vi "Omniax_mDrive_R_2016.vi"() -> ()   [LabVIEW 2014]
uses:
  <vilib>/Utility/file.llb/Read From Spreadsheet File (I64).vi
  <vilib>/Utility/file.llb/Read From Spreadsheet File (string).vi
  <vilib>/Instr/_visa.llb/VISA Configure Serial Port (Instr).vi
  <vilib>/Utility/file.llb/Write To Spreadsheet File (I64).vi
  <vilib>/Utility/file.llb/Write To Spreadsheet File (string).vi
panel:
  in  "R Move Set":bool
  in  "SSE:OmniaxR.SV":dbl
  in  "X Position SP mm":dbl
  in  "X Velocity SP mm/sec":dbl
  in  "X Move Set":bool
  in  "Y Move Set":bool
  in  "Y Position SP mm":dbl
  in  "Y Velocity SP mm/sec":dbl
  in  "Z Position SP mm":dbl
  in  "Z Velocity SP mm/sec":dbl
  in  "Z Move Set":bool
  in  "Reset Y Position mm":dbl
  out "Reset Y Motor Steps":i32
  in  "Reset X Position mm":dbl
  out "Reset X Motor Steps":i32
  in  "Reset Z Position mm":dbl
  out "Reset Z Motor Steps":i32
  in  "Submit":bool
  in  "ELOG":string
  out "Z max step":i32
  in  "V5 position 15360000":i32
  out "R Velocity MVdeg/sec":dbl format="%.3f"
  out "R Position MV deg":dbl
  out "Z Velocity MV mm/sec":dbl format="%.3f"
  out "Z Position MV mm":dbl
  out "Y Velocity MV mm/sec":dbl format="%.3f"
  out "Y Position MV mm":dbl
  out "X Velocity MV mm/sec":dbl format="%.3f"
  out "X Position MV mm":dbl
  out "Presets":i32[][](array[numeric])
  in  "stop":bool
  in  "Tab Control 3":enum32{"Status", "Reset"}(tab)
  out "R in Range":bool
  out "R Scan":bool
  out "R in Motion":bool
  out "R Backlash corr":bool
  out "R Ready":bool
  in  "Reset R Position deg":dbl
  out "Reset R Motor Steps":i32
  in  "Reset":bool
  in  "Tab Control 2":enum32{"mm", "step"}(tab)
  in  "X Scan Length SP mm":dbl
  in  "X Scan Velocity SP mm/sec":dbl
  in  "X Scan set":bool
  in  "Y Scan Length SP mm":dbl
  in  "Y Scan Velocity SP mm/sec":dbl
  in  "Y Scan set":bool
  in  "Z Scan Length SP mm":dbl
  in  "Z Scan Velocity SP mm/sec":dbl
  in  "Z Scan set":bool
  in  "R Scan Length SP deg":dbl
  in  "R Scan Velocity SP deg/sec":dbl
  in  "R Scan set":bool
  in  "X Scan Velocity SP steps/sec":i32=1 min=1 max=102400 step=1
  in  "X Scan Length SP steps":i32 min=-2816000 max=1792000 step=100
  out "X Scan length MV mm":dbl
  out "X Scan velocity MV mm/sec":dbl format="%#_6f"
  in  "Y Scan Velocity SP steps/sec":i32=1 min=1 max=102400 step=1
  in  "Y Scan Length SP steps":i32 min=-1930240 max=2677760 step=100
  out "Y Scan length MV mm":dbl
  out "Y Scan velocity MV mm/sec":dbl format="%#_6f"
  in  "Z Scan Velocity SP steps/sec":i32=1 min=1 max=102400 step=1
  in  "Z Scan Length SP steps":i32 min=-91980800 max=10419200 step=100
  out "Z Scan length MV mm":dbl
  out "Z Scan velocity MV mm/sec":dbl format="%#_6f"
  in  "R Scan Velocity SP steps/sec":i32=1 min=1 max=102400 step=1
  in  "R Scan Length SP steps":i32 min=-1501867 max=10786133 step=100
  out "R Scan length MV deg":dbl
  out "R Scan velocity MV deg/sec":dbl format="%#_6f"
  out "atan Y/Z":dbl
  in  "Tab Control":enum32{"mm", "preset", "step"}(tab)
  in  "R Velocity SP deg/sec":dbl
  in  "Add Button":bool
  in  "String":string
  in  "Delete Button":bool
  in  "Preset positions":i32(ring) items=["ZERO", "Default", "CDOSE", "QMS", "test", "test2", "test3", "yag position", "Sample Long Edge  ", "SPUTTER POS"]
  in  "Set Button":bool
  in  "X Velocity SP step/sec":i32 min=1 max=128000
  in  "Y Velocity SP step/sec":i32 min=1 max=128000
  in  "Z Velocity SP step/sec":i32 min=1 max=204800
  in  "R Velocity SP step/sec":i32 min=1 max=10000
  in  "Y Step SP":i32=-20000 min=-2304000 max=2304000 step=500
  in  "X Step SP":i32=-20000 min=-2304000 max=2304000 step=500
  in  "Z Step SP":i32=-20000 min=0 max=102400000 step=500
  in  "R Step SP":i32=-20000 min=-61440000 max=61440000 step=500
  out "X Step PV":i32 max=2000
  out "Y Step PV":i32 max=2000
  out "Z Step PV":i32 max=2000
  out "R Step PV":i32 max=2000
  in  "Clear ZY":bool
  out "X Scan Duration":dbl
  out "Y Scan Duration":dbl
  out "Z Scan Duration":dbl
  out "R Scan Duration":dbl
  out "R Backlash steps/sec":i32
  out "R Backlash":i32
  out "R Holding Current %":i32
  out "R Run Current %":i32
  out "R offset deg":dbl
  out "R deg/rev":dbl
  out "R steps/rev":u32
  out "R velocity PV step/sec":i32
  out "R MINPOS":i32=-94296
  out "R MAXPOS":i32=-34296
  out "R COM PORT":refnum<visa-resource-name>="COM5"
  in  "R Scan OK":bool
  in  "R Go":bool
  out "R Position deg PV":dbl
  out "Z Backlash steps/sec":i32
  out "Z Backlash":i32
  out "Z Holding Current %":i32
  out "Z Run Current %":i32
  out "Z offset mm":dbl
  out "Z mm/rev":dbl
  out "Z steps/rev":u32
  out "Z  velocity PV step/sec":i32
  in  "Z Scan OK":bool
  in  "Z Go":bool
  out "Z Position mm PV":dbl
  out "X Position mm PV":dbl
  out "X velocity PV step/sec":i32
  in  "X Scan OK":bool
  in  "X Go":bool
  out "X Backlash steps/sec":i32
  out "X Backlash":i32
  out "X Holding Current %":i32
  out "X Run Current %":i32
  out "X offset mm":dbl
  out "X mm/rev":dbl
  out "X steps/rev":u32
  out "Y Backlash steps/sec":i32
  out "Y Backlash":i32
  out "Y Holding Current %":i32
  out "Y Run Current %":i32
  in  "Scan Cancel":bool
  out "Y Position mm PV":dbl
  out "Y offset mm":dbl
  out "Y mm/rev":dbl
  out "Y steps/rev":u32
  out "Y velocity PV step/sec":i32
  in  "Y Scan OK":bool
  in  "Scan Go":bool
  in  "Stop":bool
  in  "Y Go":bool
  # "COM13"
  # "Goto position"
  # "SSE:OmniaxR.RV"
  # "R"
  # "MX"
  # "MR"
  # "MY"
  # "MZ"
  # "L"
  # "M"
  # "B"
  # "S"
  # "R"
  # "Preset position"
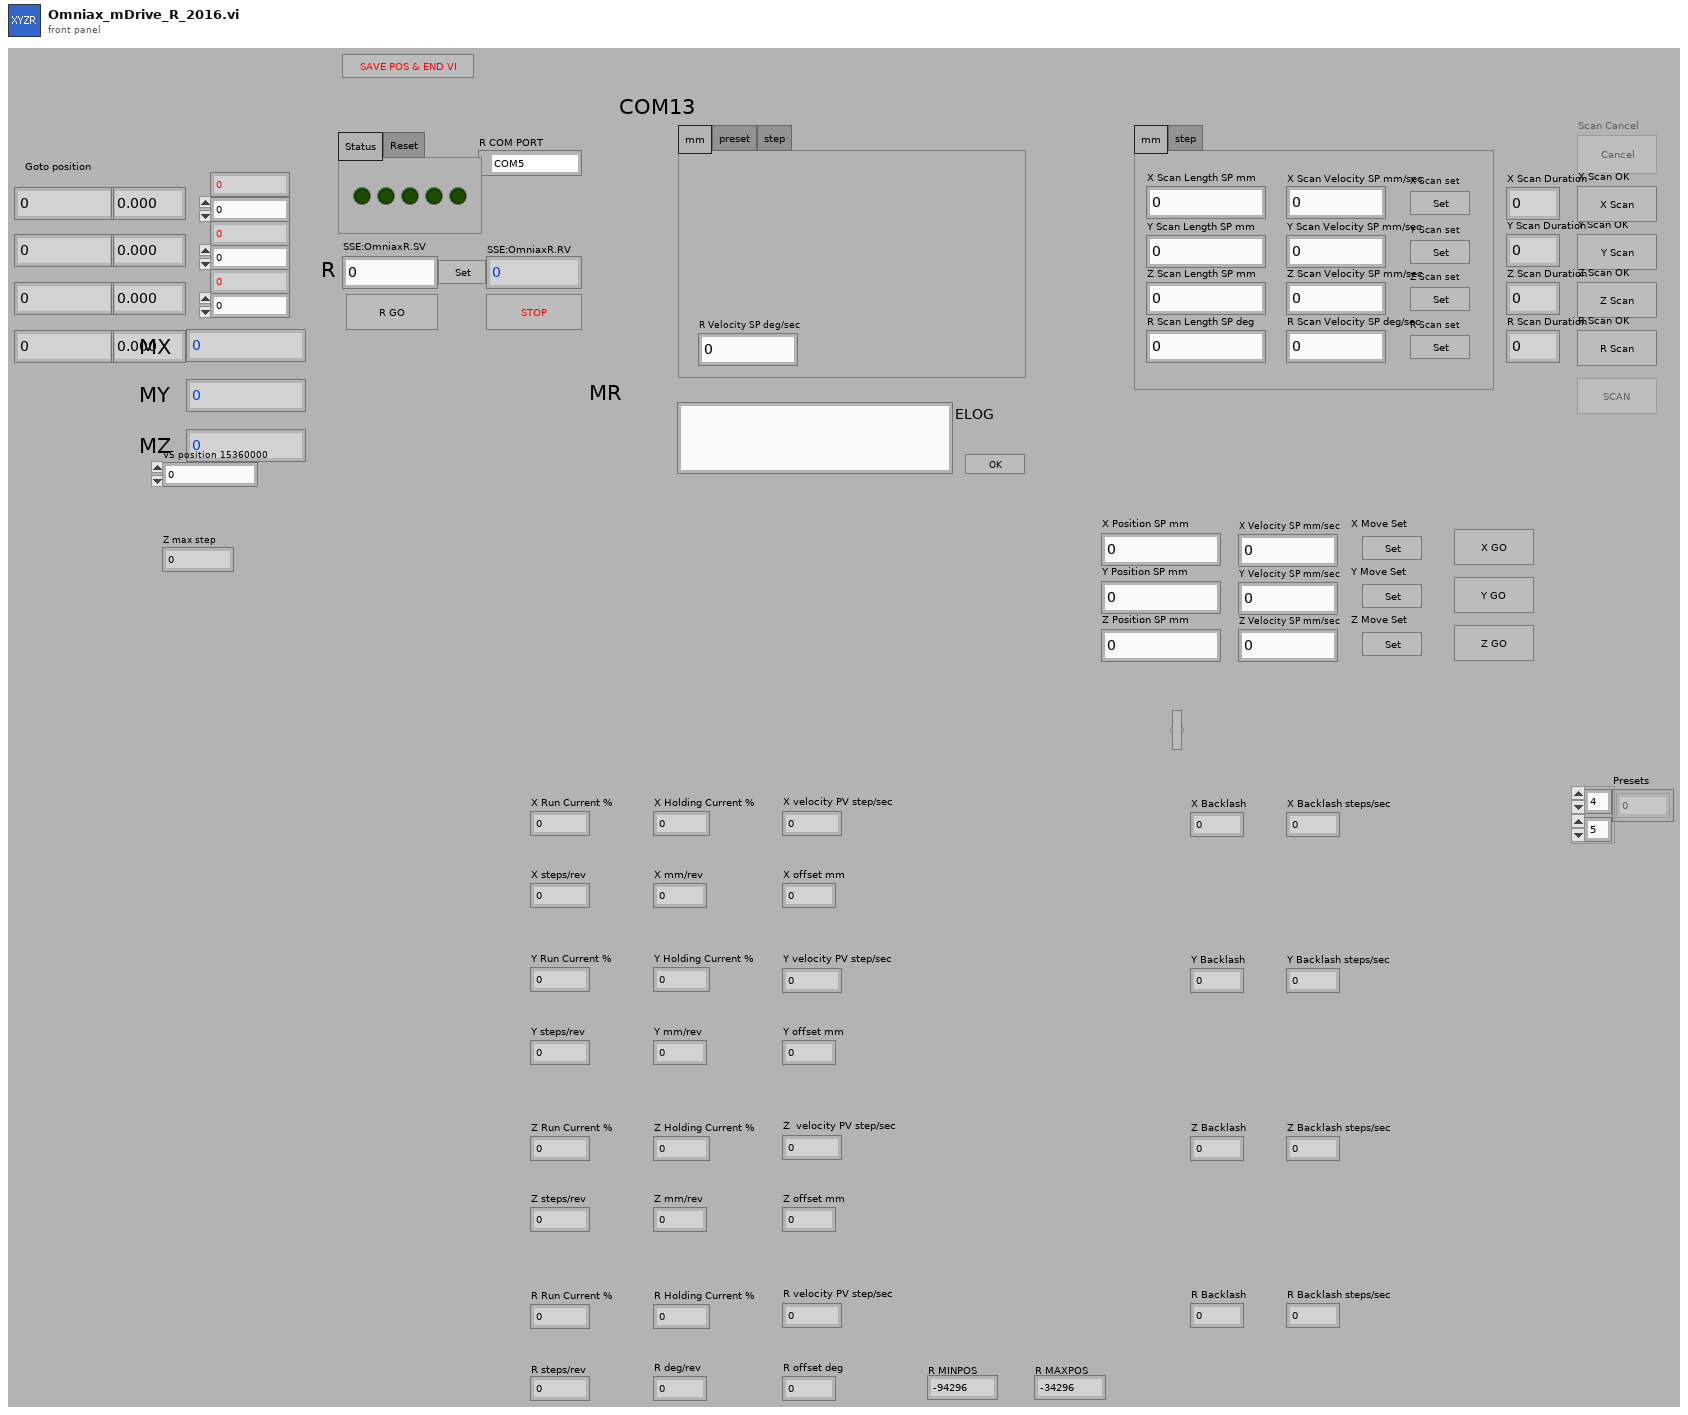
[diagram p1: front panel]
types:
  T1 = enum16{"Stop", "Reset", "Run Current", "Holding Current", "Accel Rate", "Decel Rate", "Move to Relative Position", "Move to Absolute Position", "Echo Mode", "Print Parameter", "Send String", "Microstep Resolution", "Set Current Position", "Max Velocity"}
  T2 = enum8{"Enabled", "Disabled", "Disabled and Grayed Out"}
  T3 = cluster{"first row[0]":i64, "first row[1]":i64, "first row[2]":i64, "first row[3]":i64, "first row[4]":i64, "first row[5]":i64, "first row[6]":i64, "first row[7]":i64, "first row[8]":i64}
  T4 = enum16{"open", "replace", "create", "open or create", "replace or create", "replace or create with confirmation"}
  T5 = cluster{"Value[0]":i32, "Value[1]":i32, "Value[2]":i32, "Value[3]":i32, "Value[4]":i32, "Value[5]":i32, "Value[6]":i32, "Value[7]":i32, "Value[8]":i32}
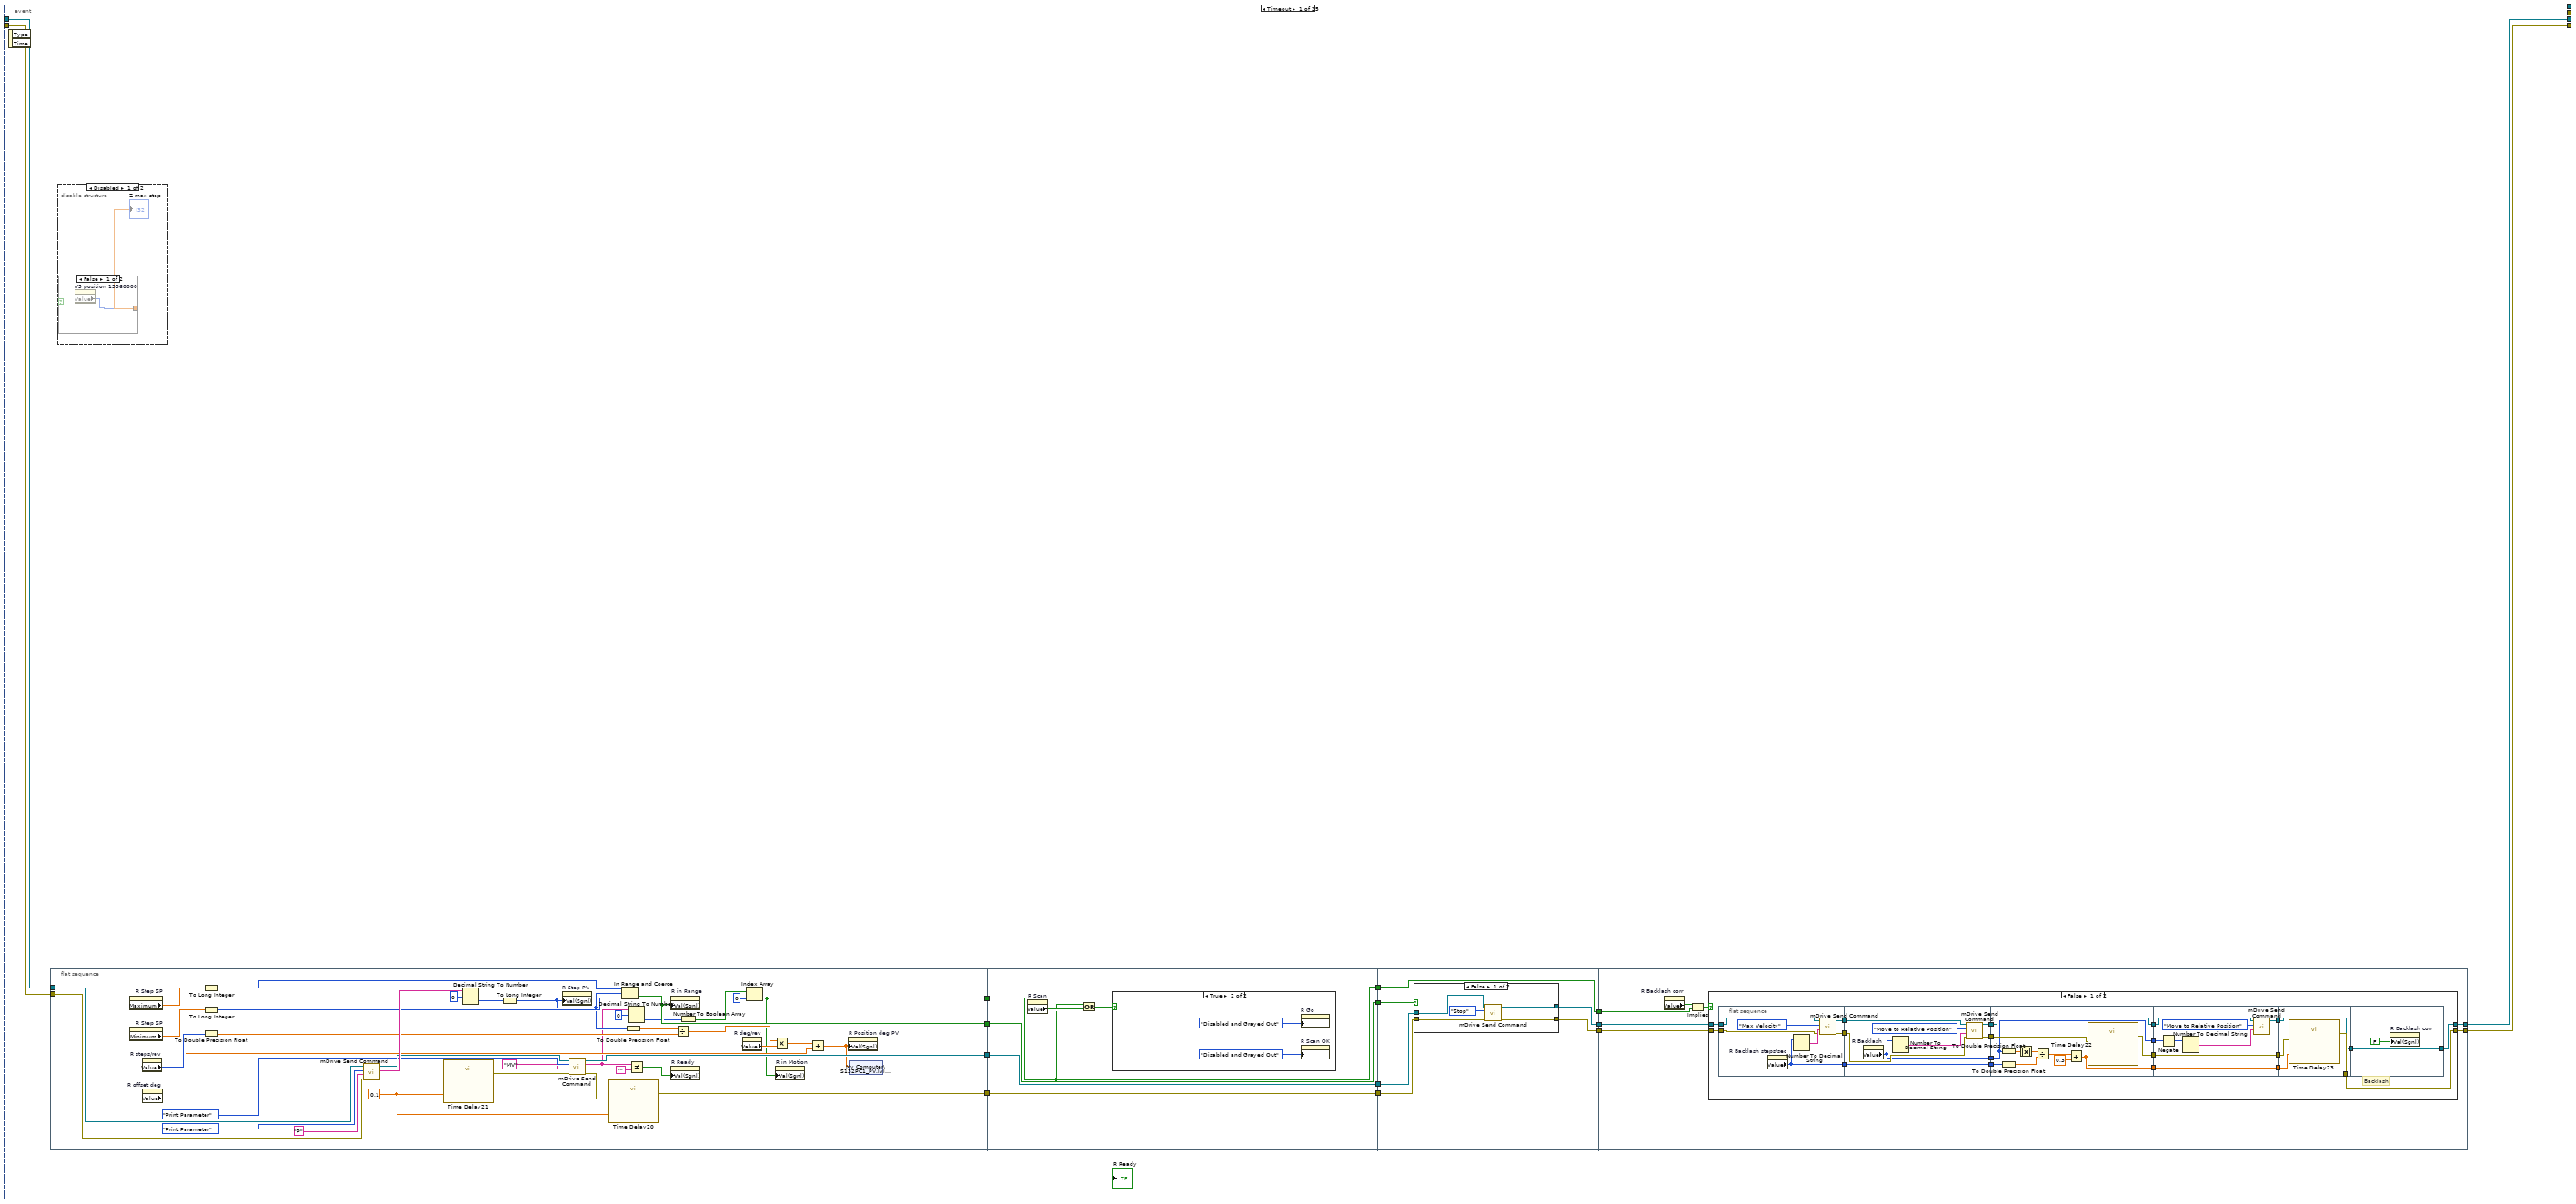
[diagram p7: hidden frame]
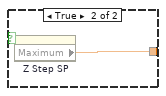
[diagram p8: hidden frame]
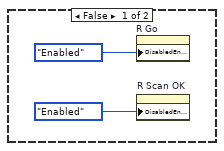
[diagram p10: hidden frame]
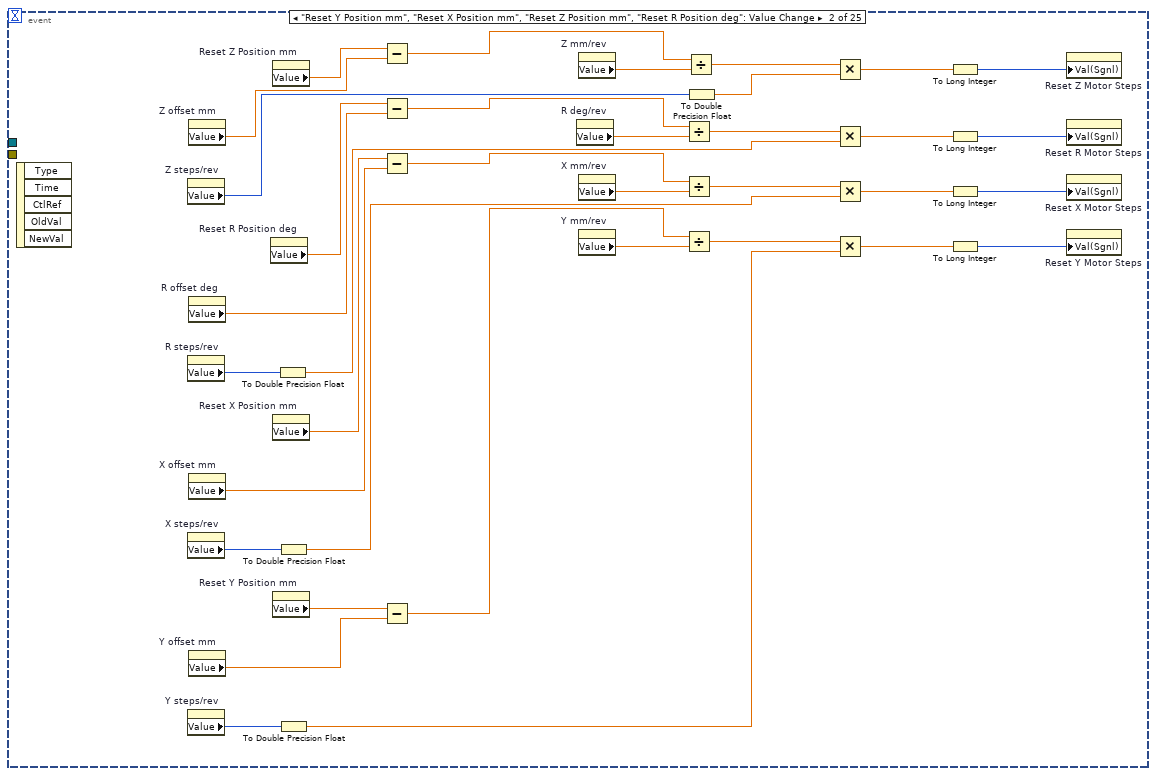
[diagram p13: hidden frame]
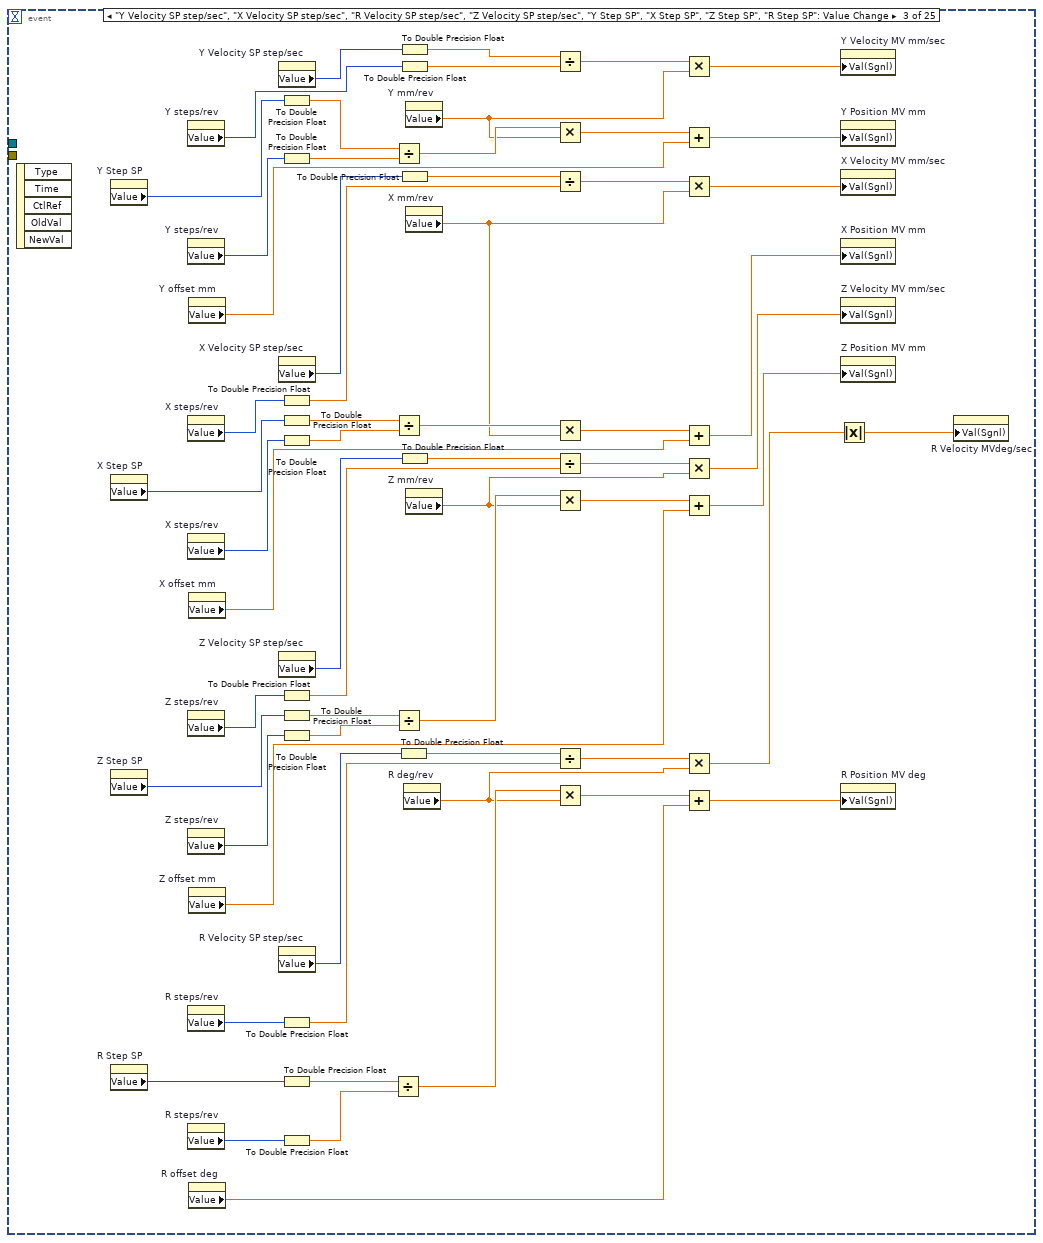
[diagram p14: hidden frame]
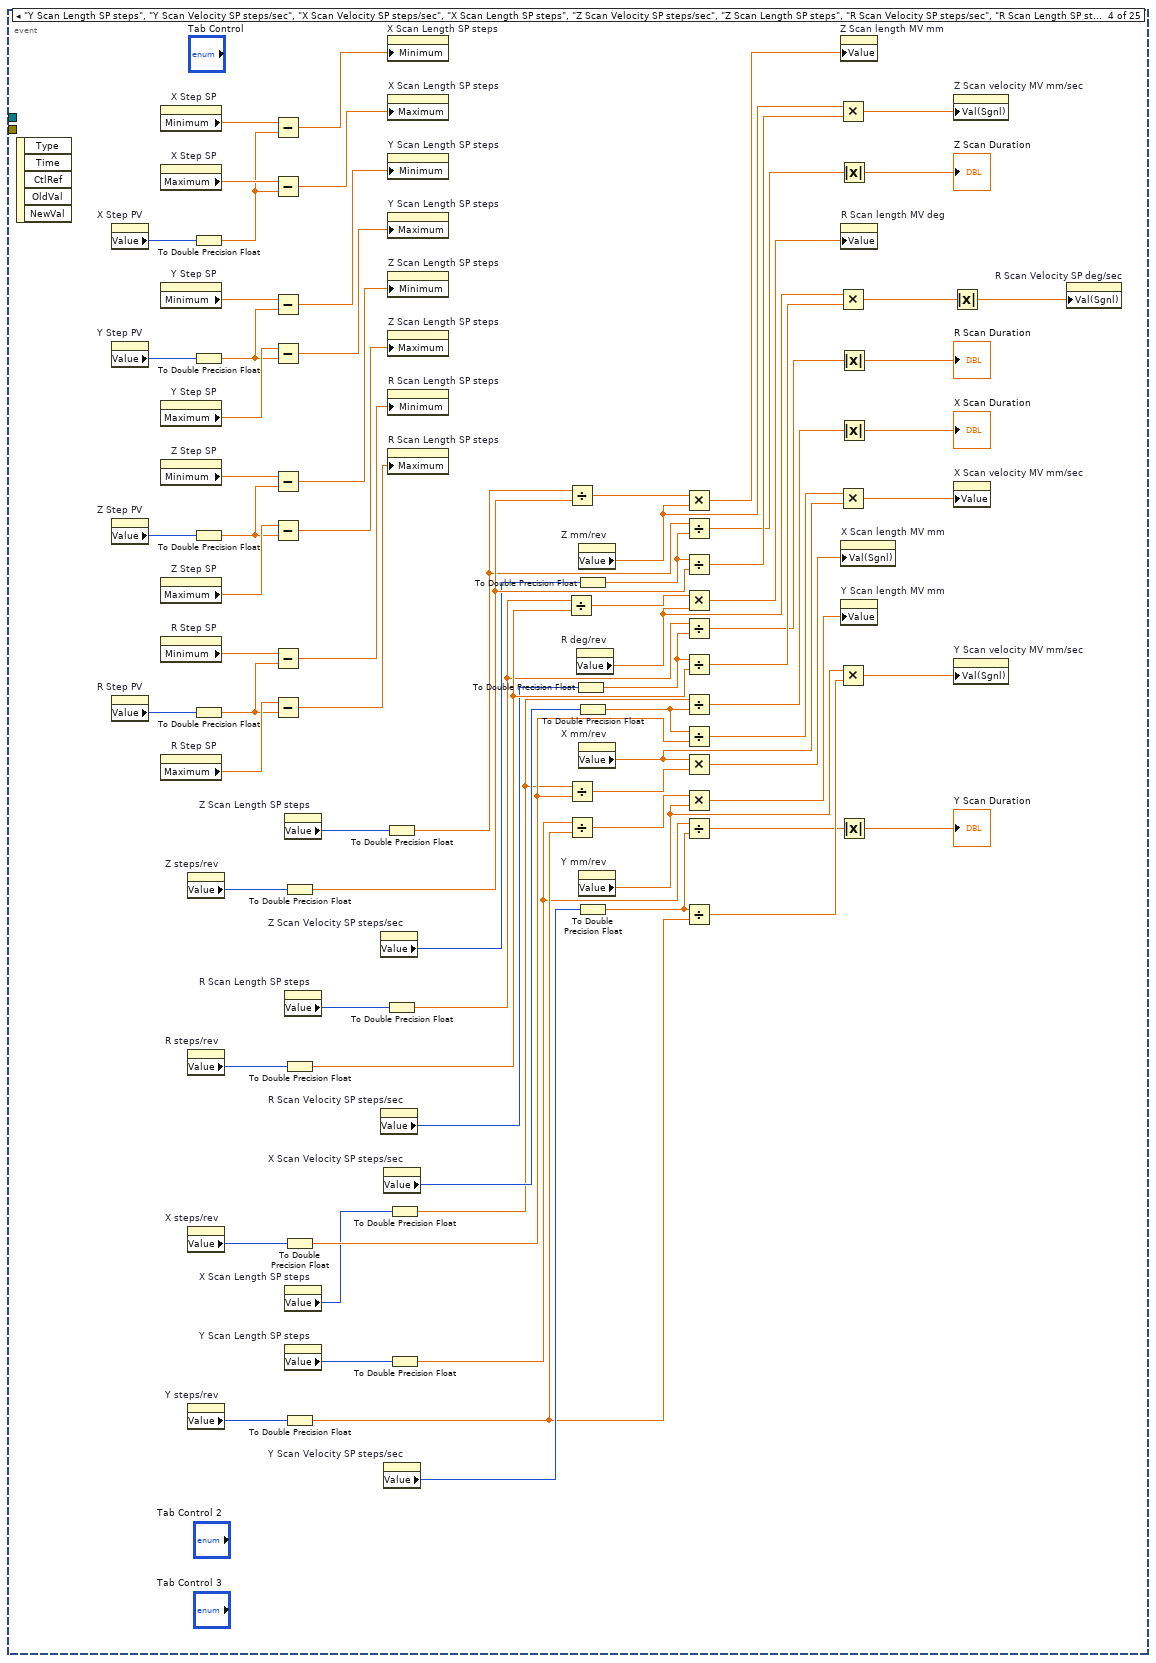
[diagram p15: hidden frame]
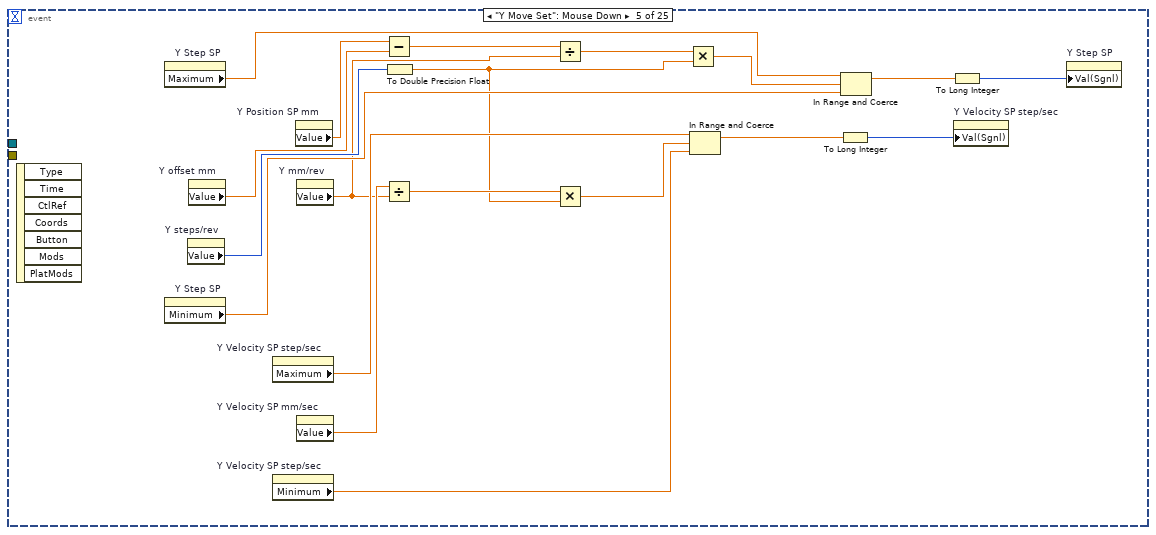
[diagram p16: hidden frame]
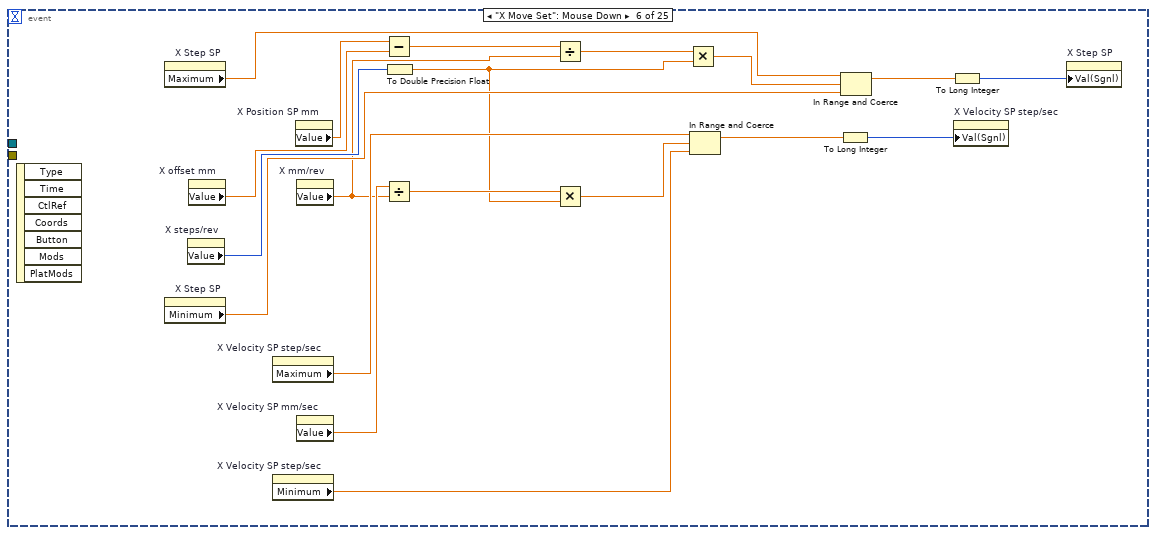
[diagram p17: hidden frame]
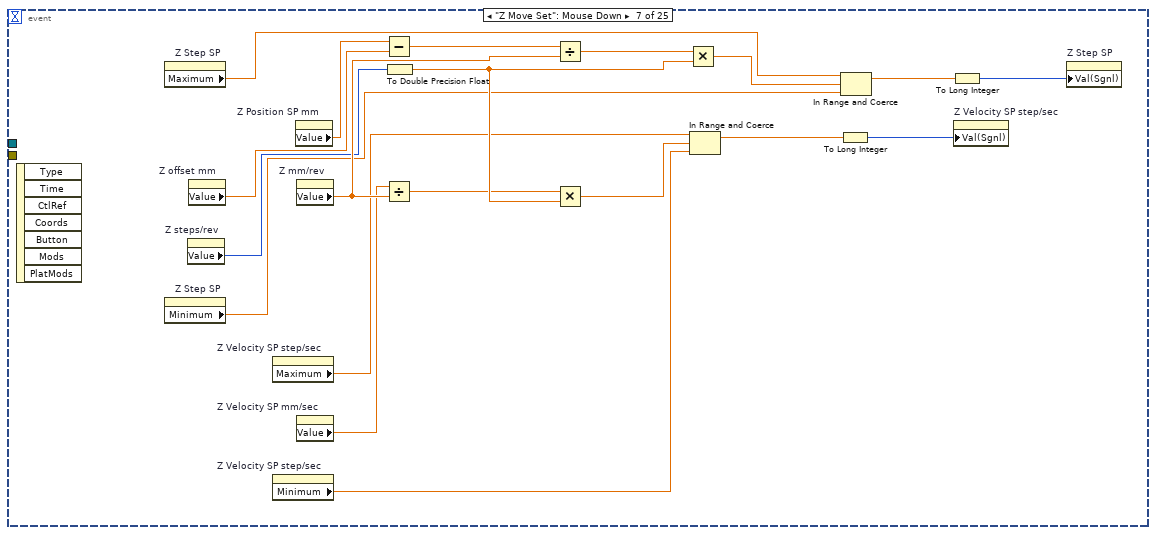
[diagram p18: hidden frame]
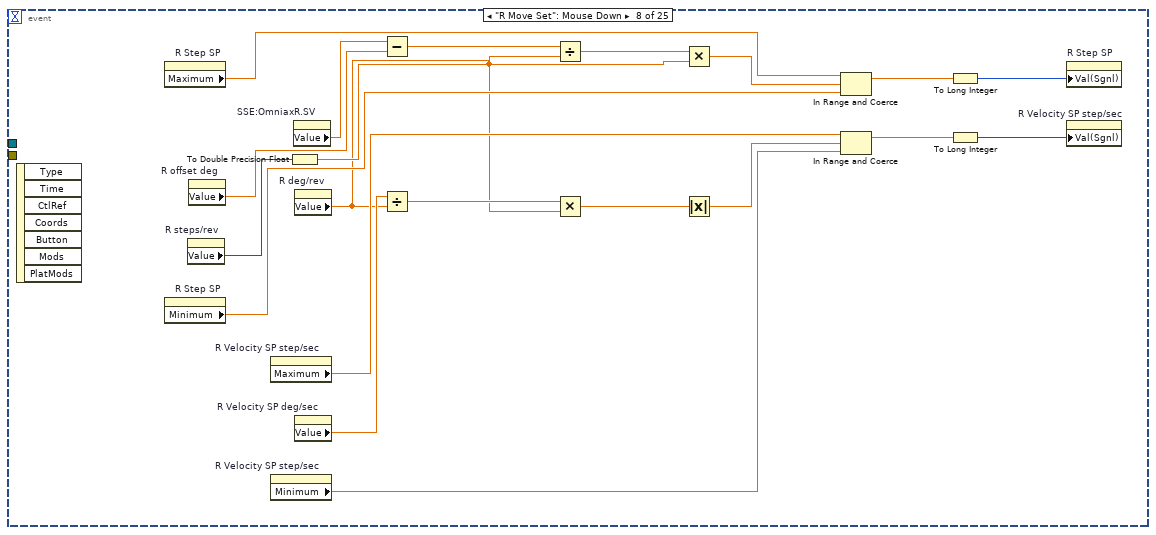
[diagram p19: hidden frame]
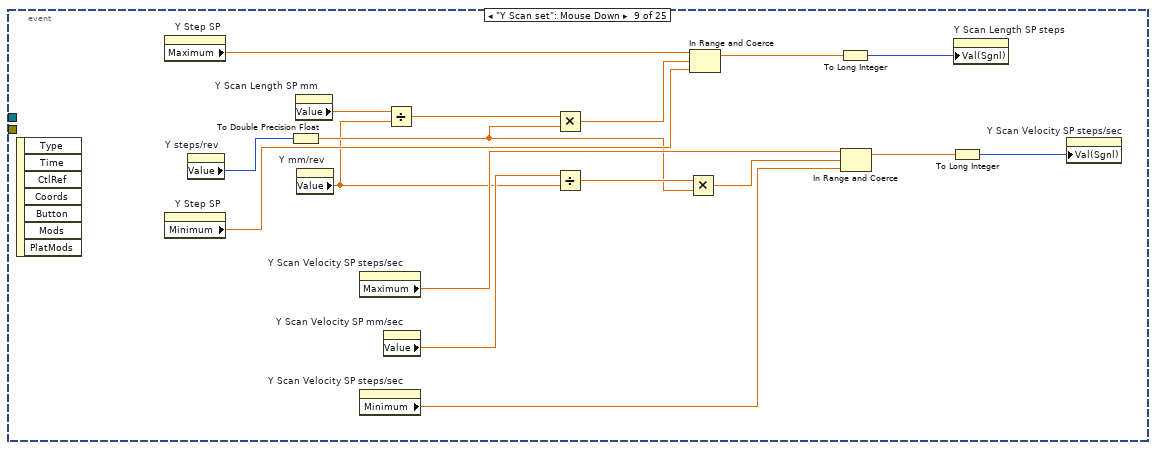
[diagram p20: hidden frame]
diagram:
  w2 = 0 ("dimension size")
  n1 = flat-sequence {
    frame #0 {
      (unwired) 6144000 ("upper limit")
      n2 = property on="R Step SP" class="DigNum (strict)"("Maximum"=61440000 ("upper limit")) -> ()  [unwired: 2 in, 2 out]
      n3 = property on="R Step SP" class="DigNum (strict)"("Minimum"=-61440000 ("lower limit")) -> ()  [unwired: 2 in, 2 out]
    }
  }
  n4 = call-poly <vilib>:"Read From Spreadsheet File.vi"("file path (dialog if empty)"=path "S:/SSE/IMS/PRESET.TXT") -> ("all rows"=w8:string[][])  [unwired: 6 in, 4 out]
  n5 = Transpose 2D Array(2D array=w8) -> (transposed array=w9:string[][])
  n6 = flat-sequence {
    tunnel: [w46] -> w25
    tunnel: [w45] -> w24
    tunnel: [w54] -> w31
    tunnel: [w56] -> w29
    tunnel: w25 -> [w55]
    tunnel: w24 -> [w57]
    tunnel: w31 -> [w61]
    tunnel: [w62] -> w30
    tunnel: w29 -> [w60]
    tunnel: [w63] -> w28
    tunnel: [w74] -> w42
    tunnel: [w76] -> w41
    tunnel: w30 -> [w75]
    tunnel: w28 -> [w70]
    tunnel: w42 -> [w83]
    tunnel: [w82] -> w40
    tunnel: w41 -> [w80]
    tunnel: [w81] -> w39
    tunnel: [w93] -> w38
    tunnel: [w94] -> w37
    tunnel: w40 -> [w92]
    tunnel: w39 -> [w91]
    tunnel: w38 -> [w104]
    tunnel: w37 -> [w103]
    tunnel: [w106] -> w36
    tunnel: [w105] -> w35
    tunnel: [w100] -> w34
    tunnel: [w113] -> w32
    tunnel: [w114] -> w33
    tunnel: w36 -> [w114]
    tunnel: w35 -> [w113]
    tunnel: w34 -> [w111]
    frame #0 {
      w53 = refnum<visa-resource-name> "COM13" ("COM PORT")
      w51 = u16 0 items=["None", "XON/XOFF", "RTS/CTS", "XON/XOFF & RTS/CTS", "DTR/DSR", "XON/XOFF & DTR/DSR"] ("flow control (0:none)")
      w50 = u16 10 items=["1.0"=10, "1.5"=15, "2.0"=20] ("stop bits (10: 1 bit)")
      # "Stop bits"
      n7 = call-poly "VISA Configure Serial Port"("VISA resource name"=w53, "timeout (10sec)"=u32 10000, "baud rate (9600)"=u32 9600, "data bits (8)"=u16 8, "parity (0:none)"=enum16{"None", "Odd", "Even", "Mark", "Space"}."None", "stop bits (10: 1 bit)"=w50, "flow control (0:none)"=w51) -> ("VISA resource name out"=w46:refnum<visa-resource-name>, "error out"=w45:errorcluster)  [unwired: 7 in]
      "R COM PORT" <- w53
    }
    frame #1 {
      n8 = call "mDrive Send Command.vi"("error in (no error)"=w57, "Extra"="EM=2", "Command"=T1."Send String", "VISA resource name"=w55) -> ("error out"=w56:errorcluster, "VISA resource name out"=w54:refnum<visa-resource-name>)  [unwired: 3 in, 1 out]
    }
    frame #2 {
      # "pr=1000000"
      n9 = Number To Decimal String(number=100000) -> (decimal integer string=w65:string)  [unwired: 1 in]
      n10 = call "mDrive Send Command.vi"("error in (no error)"=w60, "Extra"=w65, "Command"=T1."Accel Rate", "VISA resource name"=w61) -> ("error out"=w64:errorcluster, "VISA resource name out"=w69:refnum<visa-resource-name>)  [unwired: 3 in, 1 out]
      n11 = call "mDrive Send Command.vi"("error in (no error)"=w64, "Extra"=w65, "Command"=T1."Decel Rate", "VISA resource name"=w69) -> ("error out"=w63:errorcluster, "VISA resource name out"=w62:refnum<visa-resource-name>)  [unwired: 3 in, 1 out]
    }
    frame #3 {
      # "Run Current %"
      n12 = property on="R Run Current %" class="DigNum (strict)"() -> ("Value"=w72:i32)  [unwired: 2 in, 2 out]
      n13 = Number To Decimal String(number=w72) -> (decimal integer string=w73:string)  [unwired: 1 in]
      n14 = call "mDrive Send Command.vi"("error in (no error)"=w70, "Extra"=w73, "Command"=T1."Run Current", "VISA resource name"=w75) -> ("error out"=w76:errorcluster, "VISA resource name out"=w74:refnum<visa-resource-name>)  [unwired: 3 in, 1 out]
    }
    frame #4 {
      # "Holding Current %"
      n15 = property on="R Holding Current %" class="DigNum (strict)"() -> ("Value"=w78:i32)  [unwired: 2 in, 2 out]
      n16 = Number To Decimal String(number=w78) -> (decimal integer string=w79:string)  [unwired: 1 in]
      n17 = call "mDrive Send Command.vi"("error in (no error)"=w80, "Extra"=w79, "Command"=T1."Holding Current", "VISA resource name"=w83) -> ("error out"=w81:errorcluster, "VISA resource name out"=w82:refnum<visa-resource-name>)  [unwired: 3 in, 1 out]
    }
    frame #5 {
      # "Print Velocity Max"
      # "Velocity Max"
      n18 = property on="R Velocity SP step/sec" class="DigNum (strict)"() -> ("Value"=w90:i32)  [unwired: 2 in, 2 out]
      n19 = Number To Decimal String(number=w90) -> (decimal integer string=w89:string)  [unwired: 1 in]
      n20 = call "mDrive Send Command.vi"("error in (no error)"=w91, "Extra"=w89, "Command"=T1."Max Velocity", "VISA resource name"=w92) -> ("error out"=w87:errorcluster, "VISA resource name out"=w97:refnum<visa-resource-name>)  [unwired: 3 in, 1 out]
      n21 = call "mDrive Send Command.vi"("error in (no error)"=w87, "Extra"="VM", "Command"=T1."Print Parameter", "VISA resource name"=w97) -> ("error out"=w94:errorcluster, "read buffer"=w95:string, "VISA resource name out"=w93:refnum<visa-resource-name>)  [unwired: 3 in]
      n22 = Decimal String To Number(string=w95, offset=0) -> (number=w88:i32)  [unwired: 1 in, 1 out]
      n23 = property on="R velocity PV step/sec" class="DigNum (strict)"("Val(Sgnl)"=w88) -> ()  [unwired: 2 in, 2 out]
    }
    frame #6 {
      # "PRINT POSITION"
      n24 = call "mDrive Send Command.vi"("error in (no error)"=w103, "Extra"="P", "Command"=T1."Print Parameter", "VISA resource name"=w104) -> ("error out"=w105:errorcluster, "read buffer"=w102:string, "VISA resource name out"=w106:refnum<visa-resource-name>)  [unwired: 3 in]
      n25 = Decimal String To Number(string=w102, offset=0) -> (number=w100:i32)  [unwired: 1 in, 1 out]
    }
    frame #7 {
      n26 = property on="R Step SP" class="DigNum (strict)"("Val(Sgnl)"=w111) -> ()  [unwired: 2 in, 2 out]
      n27 = property on="R Step SP" class="DigNum (strict)"() -> ("Maximum"=w110:dbl)  [unwired: 2 in, 2 out]
      n28 = property on="R Step SP" class="DigNum (strict)"() -> ("Minimum"=w109:dbl)  [unwired: 2 in, 2 out]
      n29 = To Long Integer(number=w110) -> (32bit integer=w107:i32)
      "R MAXPOS" <- w107
      n30 = To Long Integer(number=w109) -> (32bit integer=w108:i32)
      "R MINPOS" <- w108
      n31 = In Range and Coerce(upper limit=w107, x=w111, lower limit=w108) -> (In Range?=w112:bool)  [unwired: 1 out]
      n32 = property on="R in Range" class="Bool (strict)"("Val(Sgnl)"=w112) -> ()  [unwired: 2 in, 2 out]
    }
  }
  n33 = flat-sequence {
    frame #0 {
      w120 = -3.0 ("R deg/rev")
      w118 = u32 51200 ("step/rev")
      w122 = 10000 ("Value (Signaling)")
      n34 = To Double Precision Float(number=w122) -> (double precision float=w124:dbl)
      n35 = To Double Precision Float(number=w118) -> (double precision float=w119:dbl)
      n36 = property on="R Velocity SP step/sec" class="DigNum (strict)"("Val(Sgnl)"=w122) -> ()  [unwired: 2 in, 2 out]
      n37 = property on="R Velocity SP step/sec" class="DigNum (strict)"("Minimum"=1.0 ("Data Entry Limits:Minimum")) -> ()  [unwired: 2 in, 2 out]
      n38 = Divide(x=w124, y=w119) -> (x/y=w123:dbl)
      n39 = property on="R Velocity SP step/sec" class="DigNum (strict)"("Maximum"=w124) -> ()  [unwired: 2 in, 2 out]
      n40 = Multiply(x=w123, y=w120) -> (x*y=w121:dbl)
      n41 = Absolute Value(x=w121) -> (abs(x)=w115:dbl)
      n42 = property on="R Velocity SP deg/sec" class="DigNum (strict)"("Val(Sgnl)"=w115) -> ()  [unwired: 2 in, 2 out]
      "R offset deg" <- 0.0 ("R offset deg")
      "R deg/rev" <- w120
      "R steps/rev" <- w118
    }
  }
  n43 = flat-sequence {
    frame #0 {
      w126 = 0.2 ("Z mm/rev")
      w125 = u32 51200 ("step/rev")
      w127 = 204800 ("Value (Signaling)")
      n44 = To Double Precision Float(number=w127) -> (double precision float=w131:dbl)
      n45 = To Double Precision Float(number=w125) -> (double precision float=w130:dbl)
      n46 = property on="Z Velocity SP step/sec" class="DigNum (strict)"("Val(Sgnl)"=w127) -> ()  [unwired: 2 in, 2 out]
      n47 = property on="Z Velocity SP step/sec" class="DigNum (strict)"("Minimum"=1.0 ("Data Entry Limits:Minimum")) -> ()  [unwired: 2 in, 2 out]
      n48 = Divide(x=w131, y=w130) -> (x/y=w128:dbl)
      n49 = property on="Z Velocity SP step/sec" class="DigNum (strict)"("Maximum"=w131) -> ()  [unwired: 2 in, 2 out]
      n50 = Multiply(x=w128, y=w126) -> (x*y=w129:dbl)
      n51 = property on="Z Velocity SP mm/sec" class="DigNum (strict)"("Val(Sgnl)"=w129) -> ()  [unwired: 2 in, 2 out]
      "Z offset mm" <- 0.0 ("Z offset mm")
      "Z mm/rev" <- w126
      "Z steps/rev" <- w125
    }
  }
  n52 = flat-sequence {
    frame #0 {
      (unwired) FALSE ("Value (Signaling)")
      n53 = property on="R Backlash corr" class="Bool (strict)"("Val(Sgnl)"=FALSE ("Value (Signaling)")) -> ()  [unwired: 2 in, 2 out]
      "Z Backlash steps/sec" <- 25600 ("Z Backlash steps/sec")
      "Z Backlash" <- -51200 ("Z Backlash")
      "X Backlash steps/sec" <- 25600 ("Value (Signaling)")
      "X Backlash" <- 10240 ("Backlash2")
      "Y Backlash" <- -10240 ("Backlash2")
      "Y Backlash steps/sec" <- 25600 ("Value (Signaling)")
      "R Backlash steps/sec" <- 6400 ("R Backlash steps/sec")
      "R Backlash" <- -12800 ("R Backlash")
    }
  }
  n54 = flat-sequence {
    frame #0 {
      "Z Holding Current %" <- 20 ("Z Holding Current %")
      "Z Run Current %" <- 40 ("Z Run Current %")
      "X Run Current %" <- 40 ("Run Current %")
      "X Holding Current %" <- 20 ("Holding Current %")
      "Y Run Current %" <- 40 ("Run Current %")
      "Y Holding Current %" <- 20 ("Holding Current %")
      "R Holding Current %" <- 15 ("R Holding Current %")
      "R Run Current %" <- 80 ("R Run Current %")
    }
  }
  n55 = flat-sequence {
    frame #0 {
      (unwired) FALSE ("Value (Signaling)")
      (unwired) FALSE ("Value (Signaling)")
      (unwired) FALSE ("Value (Signaling)")
      n56 = property on="X Scan Velocity SP mm/sec" class="DigNum (strict)"("Val(Sgnl)"=0.1 ("Value (Signaling)")) -> ()  [unwired: 2 in, 2 out]
      n57 = property on="Z Scan Velocity SP mm/sec" class="DigNum (strict)"("Val(Sgnl)"=0.1 ("Value (Signaling)")) -> ()  [unwired: 2 in, 2 out]
      n58 = property on="R Velocity SP deg/sec" class="DigNum (strict)"("Val(Sgnl)"=0.1 ("Value (Signaling)")) -> ()  [unwired: 2 in, 2 out]
      n59 = property on="R Scan" class="Bool (strict)"("Val(Sgnl)"=FALSE ("Value (Signaling)")) -> ()  [unwired: 2 in, 2 out]
      n60 = property on="Y Scan Velocity SP mm/sec" class="DigNum (strict)"("Val(Sgnl)"=0.1 ("Value (Signaling)")) -> ()  [unwired: 2 in, 2 out]
      n61 = property on="Scan Go" class="Bool"("DisabledEnum"=T2."Disabled and Grayed Out" ("Disabled")) -> ()  [unwired: 2 in, 2 out]
      n62 = property on="Scan Cancel" class="Bool"("DisabledEnum"=T2."Disabled and Grayed Out" ("Disabled")) -> ()  [unwired: 2 in, 2 out]
    }
  }
  n63 = flat-sequence {
    frame #0 {
      w160 = 0.2 ("MM/rev")
      w163 = u32 51200 ("step/rev")
      w158 = 128000 ("Value (Signaling)")
      # "a=1000000"
      n64 = property on="X Velocity SP step/sec" class="DigNum (strict)"("Minimum"=1.0 ("Data Entry Limits:Minimum")) -> ()  [unwired: 2 in, 2 out]
      n65 = To Double Precision Float(number=w158) -> (double precision float=w164:dbl)
      n66 = To Double Precision Float(number=w163) -> (double precision float=w162:dbl)
      n67 = property on="X Velocity SP step/sec" class="DigNum (strict)"("Val(Sgnl)"=w158) -> ()  [unwired: 2 in, 2 out]
      n68 = Divide(x=w164, y=w162) -> (x/y=w159:dbl)
      n69 = property on="X Velocity SP step/sec" class="DigNum (strict)"("Maximum"=w164) -> ()  [unwired: 2 in, 2 out]
      n70 = Multiply(x=w159, y=w160) -> (x*y=w161:dbl)
      n71 = property on="X Velocity SP mm/sec" class="DigNum (strict)"("Val(Sgnl)"=w161) -> ()  [unwired: 2 in, 2 out]
      "X offset mm" <- 0.0 ("offset")
      "X steps/rev" <- w163
      "X mm/rev" <- w160
    }
  }
  n72 = flat-sequence {
    frame #0 {
      w169 = 0.2 ("MM/rev")
      w172 = u32 51200 ("step/rev")
      w167 = 128000 ("Value (Signaling)")
      n73 = To Double Precision Float(number=w167) -> (double precision float=w173:dbl)
      n74 = To Double Precision Float(number=w172) -> (double precision float=w171:dbl)
      n75 = property on="Y Velocity SP step/sec" class="DigNum (strict)"("Minimum"=1.0 ("Data Entry Limits:Minimum")) -> ()  [unwired: 2 in, 2 out]
      n76 = property on="Y Velocity SP step/sec" class="DigNum (strict)"("Val(Sgnl)"=w167) -> ()  [unwired: 2 in, 2 out]
      n77 = Divide(x=w173, y=w171) -> (x/y=w168:dbl)
      n78 = property on="Y Velocity SP step/sec" class="DigNum (strict)"("Maximum"=w173) -> ()  [unwired: 2 in, 2 out]
      n79 = Multiply(x=w168, y=w169) -> (x*y=w170:dbl)
      n80 = property on="Y Velocity SP mm/sec" class="DigNum (strict)"("Val(Sgnl)"=w170) -> ()  [unwired: 2 in, 2 out]
      "Y offset mm" <- 0.0 ("offset")
      "Y steps/rev" <- w172
      "Y mm/rev" <- w169
    }
  }
  n81 = property on="Z Step SP" class="DigNum (strict)"("Minimum"=0 ("lower limit")) -> ()  [unwired: 2 in, 2 out]
  n82 = Delete From Array(array=w9, index (row)=0) -> (deleted portion=w10:string[], array with subset deleted=w12:string[][])  [unwired: 2 in]
  n83 = property on="Z Step SP" class="DigNum (strict)"("Maximum"=102400000 ("upper limit")) -> ()  [unwired: 2 in, 2 out]
  n84 = Transpose 2D Array(2D array=w12) -> (transposed array=w13:string[][])
  n85 = property on="Preset positions" class="Ring (strict)"("Strings []"=w10) -> ()  [unwired: 2 in, 2 out]
  n86 = Decimal String To Number(string=w13) -> (number=w11:i32[][])  [unwired: 2 in, 1 out]
  n87 = Initialize Array(w2, w2, 4 ("dimension size")) -> (w5:i32[][])
  n88 = call-poly <vilib>:"Read From Spreadsheet File.vi"("file path (dialog if empty)"=path "S:/SSE/IMS/POS.TXT") -> ("first row"=w20:i64[])  [unwired: 6 in, 4 out]
  n89 = Build Array (concatenate)(w5, w11) -> (→"Presets":i32[][])
  n90 = Array To Cluster(array=w20) -> (cluster=w19:T3)
  n91 = Unbundle(w19) -> ("first row[0]"=w17:i64, "first row[1]"=w16:i64, "first row[2]"=w15:i64, "first row[3]"=w14:i64)  [unwired: 5 out]
  n92 = property on="Reset X Motor Steps" class="DigNum (strict)"("Val(Sgnl)"=w17) -> ()  [unwired: 2 in, 2 out]
  n93 = property on="Reset Y Motor Steps" class="DigNum (strict)"("Val(Sgnl)"=w16) -> ()  [unwired: 2 in, 2 out]
  n94 = property on="Reset Z Motor Steps" class="DigNum (strict)"("Val(Sgnl)"=w15) -> ()  [unwired: 2 in, 2 out]
  n95 = property on="Reset R Motor Steps" class="DigNum (strict)"("Val(Sgnl)"=w14) -> ()  [unwired: 2 in, 2 out]
  n96 = property on="V5 position 15360000" class="DigNum (strict)"("Value"=15360000 ("V5 position 15360000")) -> ()  [unwired: 2 in, 2 out]
  n97 = while {
    tunnel: w33 -> [w187]
    tunnel: w32 -> [w186]
    tunnel: [w185] -> w23
    tunnel: [w184] -> w22
    stop <- "stop" stop-if-true
    n98 = property on="Preset positions" class="Ring (strict)"() -> ("Strings []"=w180:string[])  [unwired: 2 in, 2 out]
    n99 = case shown="True" "Submit" {
      tunnel: "ELOG" -> [_ w192]
      frame False {
      }
      frame True {
        n100 = Open/Create/Replace File(file path (use dialog)=path "S:/ELOG/SSE.LOG", operation (0:open)=T4."replace or create") -> (refnum out=w189:refnum<file>)  [unwired: 4 in, 2 out]
        n101 = flat-sequence {
          tunnel: w189 -> [w209]
          tunnel: w192 -> [w196]
          frame #0 {
            n102 = property on="R Position deg PV" class="DigNum (strict)"() -> ("Value"=w194:dbl)  [unwired: 2 in, 2 out]
            n103 = Number To Fractional String(number=w194) -> (F-format string=w193:string)  [unwired: 3 in]
            n104 = property on="X Position mm PV" class="DigNum (strict)"() -> ("Value"=w206:dbl)  [unwired: 2 in, 2 out]
            n105 = property on="Y Position mm PV" class="DigNum (strict)"() -> ("Value"=w205:dbl)  [unwired: 2 in, 2 out]
            n106 = property on="Z Position mm PV" class="DigNum (strict)"() -> ("Value"=w204:dbl)  [unwired: 2 in, 2 out]
            n107 = Number To Fractional String(number=w206) -> (F-format string=w202:string)  [unwired: 3 in]
            n108 = Number To Fractional String(number=w205) -> (F-format string=w200:string)  [unwired: 3 in]
            n109 = Number To Fractional String(number=w204) -> (F-format string=w198:string)  [unwired: 3 in]
            n110 = Concatenate Strings("MX=" ("string"), w202, " MY=" ("string"), w200, " MZ=" ("string"), w198, " MR= " ("string"), w193, " > " ("string"), w196) -> (w208:string)
            n111 = Write to Text File(file (use dialog)=w209, text=w208) -> (refnum out=w207:refnum<file>)  [unwired: 2 in, 2 out]
            n112 = Close File(refnum=w207) -> ()  [unwired: 1 in, 2 out]
          }
          frame #1 {
            n113 = disable-structure shown="Disabled" {
              frame Disabled {
                n114 = call <vilib>:"System Exec.vi"("working directory"=path "S:/ELOG", "command line"="S:\\elog\\elog.exe -h bl132pc -p 8080 -l \"BL13-2 SSE\" -w beam$2012 -s -a Type=\"Log ES setting\" -a Author=\"Omniax L\" -a Subject=\"Note\" -m SSE.LOG") -> ()  [unwired: 6 in, 4 out]
              }
              frame Enabled {
              }
            }
          }
        }
      }
    }
    n115 = event shown="[24] \"Reset\": Mouse Down" {
      selector: _ -> [_ _ _ _ _ _ _ _ _ _ _ _ _ _ _ _ _ _ _ _ _ _ _ _ _]
      dyn-events: _ -> [_ _ _ _ _ _ _ _ _ _ _ _ _ _ _ _ _ _ _ _ _ _ _ _ _]
      timeout: 100 -> [_ _ _ _ _ _ _ _ _ _ _ _ _ _ _ _ _ _ _ _ _ _ _ _ _]
      tunnel: [_ _ _ _ _ _ _ _ _ _ _ _ w706 _ _ _ _ w888 _ _ _ w983 w1017 _ _] -> _
      tunnel: [_ _ _ _ _ _ _ _ _ _ _ _ w707 _ _ _ _ w885 _ _ _ w984 w1018 _ _] -> _
      tunnel: [_ _ _ _ _ _ _ _ _ _ _ _ _ _ _ w822 w857 _ _ _ _ w982 w1010 _ _] -> _
      tunnel: [_ _ _ _ _ _ _ _ _ _ _ _ _ _ _ w821 w856 _ _ _ _ w981 w1009 _ _] -> _
      tunnel: [_ _ _ _ _ _ _ _ _ _ _ _ _ w735 _ _ _ _ w912 _ _ w980 w1006 _ w1134] -> _
      tunnel: [_ _ _ _ _ _ _ _ _ _ _ _ _ w736 _ _ _ _ w913 _ _ w979 w1005 _ w1133] -> _
      tunnel: w187 -> [w238 _ _ _ _ _ _ _ _ _ _ _ _ _ w771 _ _ _ _ w944 _ w978 w1002 w1068 w1136]
      tunnel: w186 -> [w237 _ _ _ _ _ _ _ _ _ _ _ _ _ w770 _ _ _ _ w943 _ w977 w1001 w1066 w1135]
      tunnel: [w236 _ _ _ _ _ _ _ _ _ _ _ _ _ w768 _ _ _ _ w942 _ w976 w1000 w1064 _] -> w185
      tunnel: [w235 _ _ _ _ _ _ _ _ _ _ _ _ _ w769 _ _ _ _ w941 _ w975 w999 w1063 _] -> w184
      event Timeout {
        n116 = event-data() -> ()  [unwired: 1 in, 2 out]
        n117 = flat-sequence {
          tunnel: [w290] -> w249
          tunnel: [w268] -> w248
          tunnel: [w279] -> w247
          tunnel: [w259] -> w246
          tunnel: w238 -> [w258]
          tunnel: w237 -> [w257]
          tunnel: w249 -> [w296]
          tunnel: [w296] -> w245
          tunnel: w248 -> [w295]
          tunnel: [w295] -> w244
          tunnel: w247 -> [w294]
          tunnel: [w294] -> w243
          tunnel: w246 -> [w291]
          tunnel: [w291] -> w242
          tunnel: w245 -> [w303]
          tunnel: [w304] -> w241
          tunnel: w244 -> [w306]
          tunnel: [w305] -> w240
          tunnel: w243 -> [w302]
          tunnel: [w301] -> w239
          tunnel: w242 -> [w301]
          tunnel: w241 -> [w316]
          tunnel: w240 -> [w317]
          tunnel: w239 -> [w319]
          tunnel: [w315] -> w235
          tunnel: [w314] -> w236
          frame #0 {
            w263 = 0.1 ("Delay Time (s)")
            n118 = property on="R Step SP" class="DigNum (strict)"() -> ("Maximum"=w281:dbl)  [unwired: 2 in, 2 out]
            n119 = property on="R Step SP" class="DigNum (strict)"() -> ("Minimum"=w283:dbl)  [unwired: 2 in, 2 out]
            n120 = property on="R steps/rev" class="DigNum (strict)"() -> ("Value"=w277:u32)  [unwired: 2 in, 2 out]
            n121 = property on="R offset deg" class="DigNum (strict)"() -> ("Value"=w273:dbl)  [unwired: 2 in, 2 out]
            n122 = To Long Integer(number=w281) -> (32bit integer=w280:i32)
            n123 = To Long Integer(number=w283) -> (32bit integer=w282:i32)
            n124 = To Double Precision Float(number=w277) -> (double precision float=w278:dbl)
            n125 = call "mDrive Send Command.vi"("error in (no error)"=w257, "Extra"="P", "Command"=T1."Print Parameter", "VISA resource name"=w258) -> ("error out"=w285:errorcluster, "read buffer"=w289:string, "VISA resource name out"=w287:refnum<visa-resource-name>)  [unwired: 3 in]
            n126 = call "Time Delay21"("error in (no error)"=w285, "Delay Time (s)"=w263) -> ("error out"=w284:errorcluster)  [unwired: 9 in]
            n127 = Decimal String To Number(string=w289, offset=0) -> (number=w270:i32)  [unwired: 1 in, 1 out]
            n128 = To Long Integer(number=w270) -> (32bit integer=w271:i32)
            n129 = property on="R Step PV" class="DigNum (strict)"("Val(Sgnl)"=w271) -> ()  [unwired: 2 in, 2 out]
            n130 = call "mDrive Send Command.vi"("error in (no error)"=w284, "Extra"="MV", "Command"=T1."Print Parameter", "VISA resource name"=w287) -> ("error out"=w286:errorcluster, "read buffer"=w254:string, "VISA resource name out"=w290:refnum<visa-resource-name>)  [unwired: 3 in]
            n131 = call "Time Delay20"("error in (no error)"=w286, "Delay Time (s)"=w263) -> ("error out"=w268:errorcluster)  [unwired: 9 in]
            n132 = In Range and Coerce(upper limit=w280, x=w271, lower limit=w282) -> (In Range?=w279:bool)  [unwired: 1 out]
            n133 = To Double Precision Float(number=w271) -> (double precision float=w272:dbl)
            n134 = Decimal String To Number(string=w254, offset=0 ("offset (0)")) -> (number=w262:i32)  [unwired: 1 in, 1 out]
            n135 = Not Equal?(x=w254, y="") -> (x != y?=w255:bool)
            n136 = property on="R in Range" class="Bool (strict)"("Val(Sgnl)"=w279) -> ()  [unwired: 2 in, 2 out]
            n137 = property on="R Ready" class="Bool (strict)"("Val(Sgnl)"=w255) -> ()  [unwired: 2 in, 2 out]
            n138 = Divide(x=w272, y=w278) -> (x/y=w276:dbl)
            n139 = Number To Boolean Array(number=w262) -> (Boolean array=w261:bool[])
            n140 = property on="R deg/rev" class="DigNum (strict)"() -> ("Value"=w275:dbl)  [unwired: 2 in, 2 out]
            n141 = Index Array(array=w261, index=0) -> (element=w259:bool)
            n142 = Multiply(x=w276, y=w275) -> (x*y=w274:dbl)
            n143 = property on="R in Motion" class="Bool (strict)"("Val(Sgnl)"=w259) -> ()  [unwired: 2 in, 2 out]
            n144 = Add(x=w274, y=w273) -> (x+y=w253:dbl)
            n145 = property on="R Position deg PV" class="DigNum (strict)"("Val(Sgnl)"=w253) -> ()  [unwired: 2 in, 2 out]
            n146 = shared-variable "My Computer\\S132PC1_PV.lvlib\\MR"(w253) -> ()  [unwired: 1 in, 1 out]
          }
          frame #1 {
            n147 = property on="R Scan" class="Bool (strict)"() -> ("Value"=w292:bool)  [unwired: 2 in, 2 out]
            n148 = Or(x=w291, y=w292) -> (x .or. y?=w293:bool)
            n149 = case shown="True" w293 {
              frame False {
                n150 = property on="R Go" class="Bool"("DisabledEnum"=T2."Enabled" ("Disabled")) -> ()  [unwired: 2 in, 2 out]
                n151 = property on="R Scan OK" class="Bool"("DisabledEnum"=T2."Enabled" ("Disabled")) -> ()  [unwired: 2 in, 2 out]
              }
              frame True {
                n152 = property on="R Go" class="Bool"("DisabledEnum"=T2."Disabled and Grayed Out" ("Disabled")) -> ()  [unwired: 2 in, 2 out]
                n153 = property on="R Scan OK" class="Bool"("DisabledEnum"=T2."Disabled and Grayed Out" ("Disabled")) -> ()  [unwired: 2 in, 2 out]
              }
            }
          }
          frame #2 {
            n154 = case shown="False" w302 {
              tunnel: w303 -> [w309 w313]
              tunnel: [w310 w313] -> w304
              tunnel: [w311 w312] -> w305
              tunnel: w306 -> [w308 w312]
              frame False {
                n155 = call "mDrive Send Command.vi"("error in (no error)"=w308, "Command"=T1."Stop", "VISA resource name"=w309) -> ("error out"=w311:errorcluster, "VISA resource name out"=w310:refnum<visa-resource-name>)  [unwired: 4 in, 1 out]
              }
              frame True {
              }
            }
          }
          frame #3 {
            n156 = property on="R Backlash corr" class="Bool (strict)"() -> ("Value"=w320:bool)  [unwired: 2 in, 2 out]
            n157 = Implies(1:w319, 2:w320) -> (0:w318:bool)
            n158 = case shown="False" w318 {
              tunnel: w317 -> [w327 w380]
              tunnel: w316 -> [w326 w381]
              tunnel: [w325 w380] -> w315
              tunnel: [w324 w381] -> w314
              frame False {
                # "Backlash"
                n159 = flat-sequence {
                  tunnel: [w342] -> w339
                  tunnel: [w344] -> w338
                  tunnel: [w343] -> w337
                  tunnel: w327 -> [w341]
                  tunnel: w326 -> [w340]
                  tunnel: w339 -> [w352]
                  tunnel: [w352] -> w336
                  tunnel: w338 -> [w351]
                  tunnel: w337 -> [w350]
                  tunnel: [w349] -> w335
                  tunnel: [w348] -> w334
                  tunnel: [w347] -> w323
                  tunnel: w336 -> [w362]
                  tunnel: w335 -> [w361]
                  tunnel: w334 -> [w359]
                  tunnel: [w360] -> w333
                  tunnel: [w359] -> w332
                  tunnel: [w358] -> w329
                  tunnel: [w357] -> w328
                  tunnel: w323 -> [w357]
                  tunnel: w333 -> [w373]
                  tunnel: w332 -> [w366]
                  tunnel: [w373] -> w331
                  tunnel: [w372] -> w330
                  tunnel: w329 -> [w372]
                  tunnel: w328 -> [w368]
                  tunnel: [w367] -> w321
                  tunnel: w331 -> [w377]
                  tunnel: w330 -> [w376]
                  tunnel: [w375] -> w325
                  tunnel: [w374] -> w322
                  tunnel: w321 -> [w374]
                  tunnel: [w379] -> w324
                  tunnel: w322 -> [w379]
                  frame #0 {
                    n160 = property on="R Backlash steps/sec" class="DigNum (strict)"() -> ("Value"=w342:i32)  [unwired: 2 in, 2 out]
                    n161 = Number To Decimal String(number=w342) -> (decimal integer string=w345:string)  [unwired: 1 in]
                    n162 = call "mDrive Send Command.vi"("error in (no error)"=w341, "Extra"=w345, "Command"=T1."Max Velocity", "VISA resource name"=w340) -> ("error out"=w343:errorcluster, "VISA resource name out"=w344:refnum<visa-resource-name>)  [unwired: 3 in, 1 out]
                  }
                  frame #1 {
                    n163 = property on="R Backlash" class="DigNum (strict)"() -> ("Value"=w347:i32)  [unwired: 2 in, 2 out]
                    n164 = Number To Decimal String(number=w347) -> (decimal integer string=w353:string)  [unwired: 1 in]
                    n165 = call "mDrive Send Command.vi"("error in (no error)"=w350, "Extra"=w353, "Command"=T1."Move to Relative Position", "VISA resource name"=w351) -> ("error out"=w349:errorcluster, "VISA resource name out"=w348:refnum<visa-resource-name>)  [unwired: 3 in, 1 out]
                  }
                  frame #2 {
                    n166 = To Double Precision Float(number=w357) -> (double precision float=w355:dbl)
                    n167 = To Double Precision Float(number=w362) -> (double precision float=w364:dbl)
                    n168 = Absolute Value(x=w355) -> (abs(x)=w356:dbl)
                    n169 = Divide(x=w356, y=w364) -> (x/y=w365:dbl)
                    n170 = Add(x=w365, y=0.3) -> (x+y=w358:dbl)
                    n171 = call "Time Delay22"("error in (no error)"=w361, "Delay Time (s)"=w358) -> ("error out"=w360:errorcluster)  [unwired: 9 in]
                  }
                  frame #3 {
                    n172 = Negate(x=w368) -> (-x=w369:i32)
                    n173 = Number To Decimal String(number=w369) -> (decimal integer string=w370:string)  [unwired: 1 in]
                    n174 = call "mDrive Send Command.vi"("Extra"=w370, "Command"=T1."Move to Relative Position", "VISA resource name"=w366) -> ("VISA resource name out"=w367:refnum<visa-resource-name>)  [unwired: 4 in, 2 out]
                  }
                  frame #4 {
                    n175 = call "Time Delay23"("error in (no error)"=w377, "Delay Time (s)"=w376) -> ("error out"=w375:errorcluster)  [unwired: 9 in]
                  }
                  frame #5 {
                    n176 = property on="R Backlash corr" class="Bool (strict)"("Val(Sgnl)"=FALSE ("Value (Signaling)")) -> ()  [unwired: 2 in, 2 out]
                  }
                }
              }
              frame True {
              }
            }
          }
        }
        n177 = disable-structure shown="Disabled" {
          frame Disabled {
            n178 = case shown="False" {
              selector: _ -> [_ _]
              tunnel: [w251 w252] -> w250
              frame False {
                n179 = property on="V5 position 15360000" class="DigNum (strict)"() -> ("Value"=w251:i32)  [unwired: 2 in, 2 out]
              }
              frame True {
                n180 = property on="Z Step SP" class="DigNum (strict)"() -> ("Maximum"=w252:dbl)  [unwired: 2 in, 2 out]
              }
            }
            "Z max step" <- w250
          }
          frame Enabled {
          }
        }
      }
      event "Reset Y Position mm", "Reset X Position mm", "Reset Z Position mm", "Reset R Position deg": Value Change {
        n181 = event-data() -> ()  [unwired: 1 in, 5 out]
        n182 = property on="Z steps/rev" class="DigNum (strict)"() -> ("Value"=w393:u32)  [unwired: 2 in, 2 out]
        n183 = property on="R steps/rev" class="DigNum (strict)"() -> ("Value"=w384:u32)  [unwired: 2 in, 2 out]
        n184 = property on="X steps/rev" class="DigNum (strict)"() -> ("Value"=w402:u32)  [unwired: 2 in, 2 out]
        n185 = property on="Y steps/rev" class="DigNum (strict)"() -> ("Value"=w411:u32)  [unwired: 2 in, 2 out]
        n186 = property on="Z offset mm" class="DigNum (strict)"() -> ("Value"=w391:dbl)  [unwired: 2 in, 2 out]
        n187 = property on="R offset deg" class="DigNum (strict)"() -> ("Value"=w382:dbl)  [unwired: 2 in, 2 out]
        n188 = property on="X offset mm" class="DigNum (strict)"() -> ("Value"=w400:dbl)  [unwired: 2 in, 2 out]
        n189 = property on="Y offset mm" class="DigNum (strict)"() -> ("Value"=w409:dbl)  [unwired: 2 in, 2 out]
        n190 = property on="Reset R Position deg" class="DigNum (strict)"() -> ("Value"=w390:dbl)  [unwired: 2 in, 2 out]
        n191 = property on="Reset Z Position mm" class="DigNum (strict)"() -> ("Value"=w399:dbl)  [unwired: 2 in, 2 out]
        n192 = property on="Reset X Position mm" class="DigNum (strict)"() -> ("Value"=w408:dbl)  [unwired: 2 in, 2 out]
        n193 = property on="Reset Y Position mm" class="DigNum (strict)"() -> ("Value"=w417:dbl)  [unwired: 2 in, 2 out]
        n194 = To Double Precision Float(number=w384) -> (double precision float=w387:dbl)
        n195 = To Double Precision Float(number=w402) -> (double precision float=w405:dbl)
        n196 = To Double Precision Float(number=w411) -> (double precision float=w414:dbl)
        n197 = Subtract(x=w399, y=w391) -> (x-y=w398:dbl)
        n198 = Subtract(x=w390, y=w382) -> (x-y=w389:dbl)
        n199 = Subtract(x=w408, y=w400) -> (x-y=w407:dbl)
        n200 = Subtract(x=w417, y=w409) -> (x-y=w416:dbl)
        n201 = property on="R deg/rev" class="DigNum (strict)"() -> ("Value"=w383:dbl)  [unwired: 2 in, 2 out]
        n202 = property on="Z mm/rev" class="DigNum (strict)"() -> ("Value"=w392:dbl)  [unwired: 2 in, 2 out]
        n203 = property on="X mm/rev" class="DigNum (strict)"() -> ("Value"=w401:dbl)  [unwired: 2 in, 2 out]
        n204 = property on="Y mm/rev" class="DigNum (strict)"() -> ("Value"=w410:dbl)  [unwired: 2 in, 2 out]
        n205 = Divide(x=w389, y=w383) -> (x/y=w388:dbl)
        n206 = Divide(x=w407, y=w401) -> (x/y=w406:dbl)
        n207 = Divide(x=w416, y=w410) -> (x/y=w415:dbl)
        n208 = Divide(x=w398, y=w392) -> (x/y=w397:dbl)
        n209 = To Double Precision Float(number=w393) -> (double precision float=w396:dbl)
        n210 = Multiply(x=w397, y=w396) -> (x*y=w395:dbl)
        n211 = Multiply(x=w388, y=w387) -> (x*y=w386:dbl)
        n212 = Multiply(x=w406, y=w405) -> (x*y=w404:dbl)
        n213 = Multiply(x=w415, y=w414) -> (x*y=w413:dbl)
        n214 = To Long Integer(number=w395) -> (32bit integer=w394:i32)
        n215 = To Long Integer(number=w386) -> (32bit integer=w385:i32)
        n216 = To Long Integer(number=w404) -> (32bit integer=w403:i32)
        n217 = To Long Integer(number=w413) -> (32bit integer=w412:i32)
        n218 = property on="Reset Z Motor Steps" class="DigNum (strict)"("Val(Sgnl)"=w394) -> ()  [unwired: 2 in, 2 out]
        n219 = property on="Reset R Motor Steps" class="DigNum (strict)"("Val(Sgnl)"=w385) -> ()  [unwired: 2 in, 2 out]
        n220 = property on="Reset X Motor Steps" class="DigNum (strict)"("Val(Sgnl)"=w403) -> ()  [unwired: 2 in, 2 out]
        n221 = property on="Reset Y Motor Steps" class="DigNum (strict)"("Val(Sgnl)"=w412) -> ()  [unwired: 2 in, 2 out]
      }
      event "Y Velocity SP step/sec", "X Velocity SP step/sec", "R Velocity SP step/sec", "Z Velocity SP step/sec", "Y Step SP", "X Step SP", "Z Step SP", "R Step SP": Value Change {
        n222 = event-data() -> ()  [unwired: 1 in, 5 out]
        n223 = property on="Y Step SP" class="DigNum (strict)"() -> ("Value"=w450:i32)  [unwired: 2 in, 2 out]
        n224 = property on="X Step SP" class="DigNum (strict)"() -> ("Value"=w442:i32)  [unwired: 2 in, 2 out]
        n225 = property on="Z Step SP" class="DigNum (strict)"() -> ("Value"=w434:i32)  [unwired: 2 in, 2 out]
        n226 = property on="R Step SP" class="DigNum (strict)"() -> ("Value"=w426:i32)  [unwired: 2 in, 2 out]
        n227 = property on="Y steps/rev" class="DigNum (strict)"() -> ("Value"=w473:u32)  [unwired: 2 in, 2 out]
        n228 = property on="Y steps/rev" class="DigNum (strict)"() -> ("Value"=w448:u32)  [unwired: 2 in, 2 out]
        n229 = property on="X steps/rev" class="DigNum (strict)"() -> ("Value"=w467:u32)  [unwired: 2 in, 2 out]
        n230 = property on="X steps/rev" class="DigNum (strict)"() -> ("Value"=w440:u32)  [unwired: 2 in, 2 out]
        n231 = property on="Z steps/rev" class="DigNum (strict)"() -> ("Value"=w461:u32)  [unwired: 2 in, 2 out]
        n232 = property on="Z steps/rev" class="DigNum (strict)"() -> ("Value"=w432:u32)  [unwired: 2 in, 2 out]
        n233 = property on="R steps/rev" class="DigNum (strict)"() -> ("Value"=w455:u32)  [unwired: 2 in, 2 out]
        n234 = property on="R steps/rev" class="DigNum (strict)"() -> ("Value"=w424:u32)  [unwired: 2 in, 2 out]
        n235 = property on="Y offset mm" class="DigNum (strict)"() -> ("Value"=w447:dbl)  [unwired: 2 in, 2 out]
        n236 = property on="X offset mm" class="DigNum (strict)"() -> ("Value"=w439:dbl)  [unwired: 2 in, 2 out]
        n237 = property on="Z offset mm" class="DigNum (strict)"() -> ("Value"=w431:dbl)  [unwired: 2 in, 2 out]
        n238 = property on="R offset deg" class="DigNum (strict)"() -> ("Value"=w423:dbl)  [unwired: 2 in, 2 out]
        n239 = property on="Y Velocity SP step/sec" class="DigNum (strict)"() -> ("Value"=w475:i32)  [unwired: 2 in, 2 out]
        n240 = property on="X Velocity SP step/sec" class="DigNum (strict)"() -> ("Value"=w469:i32)  [unwired: 2 in, 2 out]
        n241 = property on="Z Velocity SP step/sec" class="DigNum (strict)"() -> ("Value"=w463:i32)  [unwired: 2 in, 2 out]
        n242 = property on="R Velocity SP step/sec" class="DigNum (strict)"() -> ("Value"=w457:i32)  [unwired: 2 in, 2 out]
        n243 = To Double Precision Float(number=w450) -> (double precision float=w451:dbl)
        n244 = To Double Precision Float(number=w448) -> (double precision float=w454:dbl)
        n245 = To Double Precision Float(number=w467) -> (double precision float=w472:dbl)
        n246 = To Double Precision Float(number=w442) -> (double precision float=w443:dbl)
        n247 = To Double Precision Float(number=w440) -> (double precision float=w446:dbl)
        n248 = To Double Precision Float(number=w461) -> (double precision float=w466:dbl)
        n249 = To Double Precision Float(number=w434) -> (double precision float=w435:dbl)
        n250 = To Double Precision Float(number=w432) -> (double precision float=w438:dbl)
        n251 = To Double Precision Float(number=w455) -> (double precision float=w460:dbl)
        n252 = To Double Precision Float(number=w426) -> (double precision float=w427:dbl)
        n253 = To Double Precision Float(number=w424) -> (double precision float=w430:dbl)
        n254 = Divide(x=w427, y=w430) -> (x/y=w429:dbl)
        n255 = Divide(x=w451, y=w454) -> (x/y=w453:dbl)
        n256 = Divide(x=w443, y=w446) -> (x/y=w445:dbl)
        n257 = Divide(x=w435, y=w438) -> (x/y=w437:dbl)
        n258 = To Double Precision Float(number=w457) -> (double precision float=w458:dbl)
        n259 = To Double Precision Float(number=w475) -> (double precision float=w476:dbl)
        n260 = To Double Precision Float(number=w473) -> (double precision float=w478:dbl)
        n261 = To Double Precision Float(number=w469) -> (double precision float=w470:dbl)
        n262 = To Double Precision Float(number=w463) -> (double precision float=w464:dbl)
        n263 = property on="R deg/rev" class="DigNum (strict)"() -> ("Value"=w422:dbl)  [unwired: 2 in, 2 out]
        n264 = property on="Y mm/rev" class="DigNum (strict)"() -> ("Value"=w419:dbl)  [unwired: 2 in, 2 out]
        n265 = property on="X mm/rev" class="DigNum (strict)"() -> ("Value"=w420:dbl)  [unwired: 2 in, 2 out]
        n266 = property on="Z mm/rev" class="DigNum (strict)"() -> ("Value"=w421:dbl)  [unwired: 2 in, 2 out]
        n267 = Divide(x=w476, y=w478) -> (x/y=w477:dbl)
        n268 = Multiply(x=w453, y=w419) -> (x*y=w452:dbl)
        n269 = Divide(x=w470, y=w472) -> (x/y=w471:dbl)
        n270 = Multiply(x=w445, y=w420) -> (x*y=w444:dbl)
        n271 = Divide(x=w464, y=w466) -> (x/y=w465:dbl)
        n272 = Multiply(x=w437, y=w421) -> (x*y=w436:dbl)
        n273 = Divide(x=w458, y=w460) -> (x/y=w459:dbl)
        n274 = Multiply(x=w429, y=w422) -> (x*y=w428:dbl)
        n275 = Multiply(x=w477, y=w419) -> (x*y=w474:dbl)
        n276 = Add(x=w452, y=w447) -> (x+y=w449:dbl)
        n277 = Multiply(x=w471, y=w420) -> (x*y=w468:dbl)
        n278 = Add(x=w444, y=w439) -> (x+y=w441:dbl)
        n279 = Multiply(x=w465, y=w421) -> (x*y=w462:dbl)
        n280 = Add(x=w436, y=w431) -> (x+y=w433:dbl)
        n281 = Multiply(x=w459, y=w422) -> (x*y=w456:dbl)
        n282 = Add(x=w428, y=w423) -> (x+y=w425:dbl)
        n283 = Absolute Value(x=w456) -> (abs(x)=w418:dbl)
        n284 = property on="Y Velocity MV mm/sec" class="DigNum (strict)"("Val(Sgnl)"=w474) -> ()  [unwired: 2 in, 2 out]
        n285 = property on="Y Position MV mm" class="DigNum (strict)"("Val(Sgnl)"=w449) -> ()  [unwired: 2 in, 2 out]
        n286 = property on="X Velocity MV mm/sec" class="DigNum (strict)"("Val(Sgnl)"=w468) -> ()  [unwired: 2 in, 2 out]
        n287 = property on="X Position MV mm" class="DigNum (strict)"("Val(Sgnl)"=w441) -> ()  [unwired: 2 in, 2 out]
        n288 = property on="Z Velocity MV mm/sec" class="DigNum (strict)"("Val(Sgnl)"=w462) -> ()  [unwired: 2 in, 2 out]
        n289 = property on="Z Position MV mm" class="DigNum (strict)"("Val(Sgnl)"=w433) -> ()  [unwired: 2 in, 2 out]
        n290 = property on="R Position MV deg" class="DigNum (strict)"("Val(Sgnl)"=w425) -> ()  [unwired: 2 in, 2 out]
        n291 = property on="R Velocity MVdeg/sec" class="DigNum (strict)"("Val(Sgnl)"=w418) -> ()  [unwired: 2 in, 2 out]
      }
      event "Y Scan Length SP steps", "Y Scan Velocity SP steps/sec", "X Scan Velocity SP steps/sec", "X Scan Length SP steps", "Z Scan Velocity SP steps/sec", "Z Scan Length SP steps", "R Scan Velocity SP steps/sec", "R Scan Length SP steps": Value Change {
        n292 = event-data() -> ()  [unwired: 1 in, 5 out]
        n293 = property on="X Step PV" class="DigNum (strict)"() -> ("Value"=w547:i32)  [unwired: 2 in, 2 out]
        n294 = property on="Y Step PV" class="DigNum (strict)"() -> ("Value"=w533:i32)  [unwired: 2 in, 2 out]
        n295 = property on="Z Step PV" class="DigNum (strict)"() -> ("Value"=w520:i32)  [unwired: 2 in, 2 out]
        n296 = property on="R Step PV" class="DigNum (strict)"() -> ("Value"=w506:i32)  [unwired: 2 in, 2 out]
        n297 = property on="X Step SP" class="DigNum (strict)"() -> ("Minimum"=w554:dbl)  [unwired: 2 in, 2 out]
        n298 = property on="X Step SP" class="DigNum (strict)"() -> ("Maximum"=w553:dbl)  [unwired: 2 in, 2 out]
        n299 = property on="Y Step SP" class="DigNum (strict)"() -> ("Minimum"=w540:dbl)  [unwired: 2 in, 2 out]
        n300 = property on="Y Step SP" class="DigNum (strict)"() -> ("Maximum"=w539:dbl)  [unwired: 2 in, 2 out]
        n301 = property on="Z Step SP" class="DigNum (strict)"() -> ("Minimum"=w527:dbl)  [unwired: 2 in, 2 out]
        n302 = property on="Z Step SP" class="DigNum (strict)"() -> ("Maximum"=w526:dbl)  [unwired: 2 in, 2 out]
        n303 = property on="R Step SP" class="DigNum (strict)"() -> ("Minimum"=w511:dbl)  [unwired: 2 in, 2 out]
        n304 = property on="R Step SP" class="DigNum (strict)"() -> ("Maximum"=w514:dbl)  [unwired: 2 in, 2 out]
        n305 = property on="Z steps/rev" class="DigNum (strict)"() -> ("Value"=w522:u32)  [unwired: 2 in, 2 out]
        n306 = property on="R steps/rev" class="DigNum (strict)"() -> ("Value"=w508:u32)  [unwired: 2 in, 2 out]
        n307 = property on="X steps/rev" class="DigNum (strict)"() -> ("Value"=w549:u32)  [unwired: 2 in, 2 out]
        n308 = property on="Y steps/rev" class="DigNum (strict)"() -> ("Value"=w535:u32)  [unwired: 2 in, 2 out]
        n309 = To Double Precision Float(number=w547) -> (double precision float=w500:dbl)
        n310 = To Double Precision Float(number=w533) -> (double precision float=w499:dbl)
        n311 = To Double Precision Float(number=w520) -> (double precision float=w498:dbl)
        n312 = To Double Precision Float(number=w506) -> (double precision float=w497:dbl)
        n313 = Subtract(x=w554, y=w500) -> (x-y=w555:dbl)
        n314 = Subtract(x=w553, y=w500) -> (x-y=w552:dbl)
        n315 = Subtract(x=w540, y=w499) -> (x-y=w541:dbl)
        n316 = Subtract(x=w539, y=w499) -> (x-y=w538:dbl)
        n317 = Subtract(x=w527, y=w498) -> (x-y=w528:dbl)
        n318 = Subtract(x=w526, y=w498) -> (x-y=w525:dbl)
        n319 = Subtract(x=w511, y=w497) -> (x-y=w512:dbl)
        n320 = Subtract(x=w514, y=w497) -> (x-y=w513:dbl)
        n321 = property on="Z Scan Length SP steps" class="DigNum (strict)"() -> ("Value"=w523:i32)  [unwired: 2 in, 2 out]
        n322 = To Double Precision Float(number=w522) -> (double precision float=w519:dbl)
        n323 = property on="R Scan Length SP steps" class="DigNum (strict)"() -> ("Value"=w509:i32)  [unwired: 2 in, 2 out]
        n324 = To Double Precision Float(number=w508) -> (double precision float=w505:dbl)
        n325 = To Double Precision Float(number=w549) -> (double precision float=w546:dbl)
        n326 = property on="X Scan Length SP steps" class="DigNum (strict)"() -> ("Value"=w545:i32)  [unwired: 2 in, 2 out]
        n327 = property on="Y Scan Length SP steps" class="DigNum (strict)"() -> ("Value"=w536:i32)  [unwired: 2 in, 2 out]
        n328 = To Double Precision Float(number=w535) -> (double precision float=w490:dbl)
        n329 = property on="Z Scan Velocity SP steps/sec" class="DigNum (strict)"() -> ("Value"=w518:i32)  [unwired: 2 in, 2 out]
        n330 = property on="R Scan Velocity SP steps/sec" class="DigNum (strict)"() -> ("Value"=w504:i32)  [unwired: 2 in, 2 out]
        n331 = property on="X Scan Velocity SP steps/sec" class="DigNum (strict)"() -> ("Value"=w550:i32)  [unwired: 2 in, 2 out]
        n332 = property on="Y Scan Velocity SP steps/sec" class="DigNum (strict)"() -> ("Value"=w532:i32)  [unwired: 2 in, 2 out]
        n333 = To Double Precision Float(number=w523) -> (double precision float=w496:dbl)
        n334 = To Double Precision Float(number=w509) -> (double precision float=w494:dbl)
        n335 = property on="X Scan Length SP steps" class="DigNum (strict)"("Minimum"=w555) -> ()  [unwired: 2 in, 2 out]
        n336 = property on="X Scan Length SP steps" class="DigNum (strict)"("Maximum"=w552) -> ()  [unwired: 2 in, 2 out]
        n337 = property on="Y Scan Length SP steps" class="DigNum (strict)"("Minimum"=w541) -> ()  [unwired: 2 in, 2 out]
        n338 = property on="Y Scan Length SP steps" class="DigNum (strict)"("Maximum"=w538) -> ()  [unwired: 2 in, 2 out]
        n339 = property on="Z Scan Length SP steps" class="DigNum (strict)"("Minimum"=w528) -> ()  [unwired: 2 in, 2 out]
        n340 = property on="Z Scan Length SP steps" class="DigNum (strict)"("Maximum"=w525) -> ()  [unwired: 2 in, 2 out]
        n341 = property on="R Scan Length SP steps" class="DigNum (strict)"("Minimum"=w512) -> ()  [unwired: 2 in, 2 out]
        n342 = property on="R Scan Length SP steps" class="DigNum (strict)"("Maximum"=w513) -> ()  [unwired: 2 in, 2 out]
        n343 = To Double Precision Float(number=w545) -> (double precision float=w485:dbl)
        n344 = To Double Precision Float(number=w536) -> (double precision float=w489:dbl)
        n345 = Divide(x=w494, y=w505) -> (x/y=w510:dbl)
        n346 = Divide(x=w496, y=w519) -> (x/y=w524:dbl)
        n347 = Divide(x=w485, y=w546) -> (x/y=w544:dbl)
        n348 = Divide(x=w489, y=w490) -> (x/y=w537:dbl)
        n349 = To Double Precision Float(number=w504) -> (double precision float=w493:dbl)
        n350 = property on="R deg/rev" class="DigNum (strict)"() -> ("Value"=w507:dbl)  [unwired: 2 in, 2 out]
        n351 = To Double Precision Float(number=w518) -> (double precision float=w495:dbl)
        n352 = To Double Precision Float(number=w550) -> (double precision float=w484:dbl)
        n353 = To Double Precision Float(number=w532) -> (double precision float=w488:dbl)
        n354 = property on="Z mm/rev" class="DigNum (strict)"() -> ("Value"=w521:dbl)  [unwired: 2 in, 2 out]
        n355 = property on="X mm/rev" class="DigNum (strict)"() -> ("Value"=w548:dbl)  [unwired: 2 in, 2 out]
        n356 = property on="Y mm/rev" class="DigNum (strict)"() -> ("Value"=w534:dbl)  [unwired: 2 in, 2 out]
        n357 = Multiply(x=w524, y=w521) -> (x*y=w516:dbl)
        n358 = Divide(x=w496, y=w495) -> (x/y=w491:dbl)
        n359 = Divide(x=w495, y=w519) -> (x/y=w517:dbl)
        n360 = Multiply(x=w510, y=w507) -> (x*y=w502:dbl)
        n361 = Divide(x=w494, y=w493) -> (x/y=w492:dbl)
        n362 = Divide(x=w493, y=w505) -> (x/y=w503:dbl)
        n363 = Divide(x=w485, y=w484) -> (x/y=w486:dbl)
        n364 = Divide(x=w484, y=w546) -> (x/y=w551:dbl)
        n365 = Multiply(x=w548, y=w544) -> (x*y=w542:dbl)
        n366 = Multiply(x=w537, y=w534) -> (x*y=w530:dbl)
        n367 = Divide(x=w489, y=w488) -> (x/y=w487:dbl)
        n368 = Divide(x=w488, y=w490) -> (x/y=w531:dbl)
        n369 = Multiply(x=w521, y=w517) -> (x*y=w515:dbl)
        n370 = Multiply(x=w507, y=w503) -> (x*y=w501:dbl)
        n371 = Multiply(x=w551, y=w548) -> (x*y=w543:dbl)
        n372 = Multiply(x=w534, y=w531) -> (x*y=w529:dbl)
        n373 = Absolute Value(x=w491) -> (abs(x)=→"Z Scan Duration":dbl)
        n374 = Absolute Value(x=w492) -> (abs(x)=→"R Scan Duration":dbl)
        n375 = Absolute Value(x=w486) -> (abs(x)=→"X Scan Duration":dbl)
        n376 = Absolute Value(x=w487) -> (abs(x)=→"Y Scan Duration":dbl)
        n377 = property on="Z Scan length MV mm" class="DigNum (strict)"("Value"=w516) -> ()  [unwired: 2 in, 2 out]
        n378 = property on="R Scan length MV deg" class="DigNum (strict)"("Value"=w502) -> ()  [unwired: 2 in, 2 out]
        n379 = property on="X Scan length MV mm" class="DigNum (strict)"("Val(Sgnl)"=w542) -> ()  [unwired: 2 in, 2 out]
        n380 = property on="Y Scan length MV mm" class="DigNum (strict)"("Value"=w530) -> ()  [unwired: 2 in, 2 out]
        n381 = Absolute Value(x=w501) -> (abs(x)=w483:dbl)
        n382 = property on="Z Scan velocity MV mm/sec" class="DigNum (strict)"("Val(Sgnl)"=w515) -> ()  [unwired: 2 in, 2 out]
        n383 = property on="X Scan velocity MV mm/sec" class="DigNum (strict)"("Value"=w543) -> ()  [unwired: 2 in, 2 out]
        n384 = property on="Y Scan velocity MV mm/sec" class="DigNum (strict)"("Val(Sgnl)"=w529) -> ()  [unwired: 2 in, 2 out]
        n385 = property on="R Scan Velocity SP deg/sec" class="DigNum (strict)"("Val(Sgnl)"=w483) -> ()  [unwired: 2 in, 2 out]
      }
      event "Y Move Set": Mouse Down {
        n386 = event-data() -> ()  [unwired: 1 in, 7 out]
        n387 = property on="Y Step SP" class="DigNum (strict)"() -> ("Maximum"=w566:dbl)  [unwired: 2 in, 2 out]
        n388 = property on="Y Step SP" class="DigNum (strict)"() -> ("Minimum"=w565:dbl)  [unwired: 2 in, 2 out]
        n389 = property on="Y steps/rev" class="DigNum (strict)"() -> ("Value"=w572:u32)  [unwired: 2 in, 2 out]
        n390 = property on="Y offset mm" class="DigNum (strict)"() -> ("Value"=w570:dbl)  [unwired: 2 in, 2 out]
        n391 = property on="Y Velocity SP step/sec" class="DigNum (strict)"() -> ("Maximum"=w559:dbl)  [unwired: 2 in, 2 out]
        n392 = property on="Y Velocity SP step/sec" class="DigNum (strict)"() -> ("Minimum"=w558:dbl)  [unwired: 2 in, 2 out]
        n393 = property on="Y Position SP mm" class="DigNum (strict)"() -> ("Value"=w569:dbl)  [unwired: 2 in, 2 out]
        n394 = property on="Y mm/rev" class="DigNum (strict)"() -> ("Value"=w556:dbl)  [unwired: 2 in, 2 out]
        n395 = property on="Y Velocity SP mm/sec" class="DigNum (strict)"() -> ("Value"=w563:dbl)  [unwired: 2 in, 2 out]
        n396 = Subtract(x=w569, y=w570) -> (x-y=w573:dbl)
        n397 = Divide(x=w563, y=w556) -> (x/y=w564:dbl)
        n398 = To Double Precision Float(number=w572) -> (double precision float=w557:dbl)
        n399 = Divide(x=w573, y=w556) -> (x/y=w574:dbl)
        n400 = Multiply(x=w564, y=w557) -> (x*y=w561:dbl)
        n401 = Multiply(x=w574, y=w557) -> (x*y=w568:dbl)
        n402 = In Range and Coerce(upper limit=w559, x=w561, lower limit=w558) -> (coerced(x)=w560:dbl)  [unwired: 1 out]
        n403 = To Long Integer(number=w560) -> (32bit integer=w562:i32)
        n404 = In Range and Coerce(upper limit=w566, x=w568, lower limit=w565) -> (coerced(x)=w567:dbl)  [unwired: 1 out]
        n405 = To Long Integer(number=w567) -> (32bit integer=w571:i32)
        n406 = property on="Y Velocity SP step/sec" class="DigNum (strict)"("Val(Sgnl)"=w562) -> ()  [unwired: 2 in, 2 out]
        n407 = property on="Y Step SP" class="DigNum (strict)"("Val(Sgnl)"=w571) -> ()  [unwired: 2 in, 2 out]
      }
      event "X Move Set": Mouse Down {
        n408 = event-data() -> ()  [unwired: 1 in, 7 out]
        n409 = property on="X Step SP" class="DigNum (strict)"() -> ("Maximum"=w585:dbl)  [unwired: 2 in, 2 out]
        n410 = property on="X Step SP" class="DigNum (strict)"() -> ("Minimum"=w584:dbl)  [unwired: 2 in, 2 out]
        n411 = property on="X steps/rev" class="DigNum (strict)"() -> ("Value"=w591:u32)  [unwired: 2 in, 2 out]
        n412 = property on="X offset mm" class="DigNum (strict)"() -> ("Value"=w589:dbl)  [unwired: 2 in, 2 out]
        n413 = property on="X Velocity SP step/sec" class="DigNum (strict)"() -> ("Maximum"=w578:dbl)  [unwired: 2 in, 2 out]
        n414 = property on="X Velocity SP step/sec" class="DigNum (strict)"() -> ("Minimum"=w577:dbl)  [unwired: 2 in, 2 out]
        n415 = property on="X Position SP mm" class="DigNum (strict)"() -> ("Value"=w588:dbl)  [unwired: 2 in, 2 out]
        n416 = property on="X mm/rev" class="DigNum (strict)"() -> ("Value"=w575:dbl)  [unwired: 2 in, 2 out]
        n417 = property on="X Velocity SP mm/sec" class="DigNum (strict)"() -> ("Value"=w582:dbl)  [unwired: 2 in, 2 out]
        n418 = Subtract(x=w588, y=w589) -> (x-y=w592:dbl)
        n419 = Divide(x=w582, y=w575) -> (x/y=w583:dbl)
        n420 = To Double Precision Float(number=w591) -> (double precision float=w576:dbl)
        n421 = Divide(x=w592, y=w575) -> (x/y=w593:dbl)
        n422 = Multiply(x=w583, y=w576) -> (x*y=w580:dbl)
        n423 = Multiply(x=w593, y=w576) -> (x*y=w587:dbl)
        n424 = In Range and Coerce(upper limit=w578, x=w580, lower limit=w577) -> (coerced(x)=w579:dbl)  [unwired: 1 out]
        n425 = To Long Integer(number=w579) -> (32bit integer=w581:i32)
        n426 = In Range and Coerce(upper limit=w585, x=w587, lower limit=w584) -> (coerced(x)=w586:dbl)  [unwired: 1 out]
        n427 = To Long Integer(number=w586) -> (32bit integer=w590:i32)
        n428 = property on="X Velocity SP step/sec" class="DigNum (strict)"("Val(Sgnl)"=w581) -> ()  [unwired: 2 in, 2 out]
        n429 = property on="X Step SP" class="DigNum (strict)"("Val(Sgnl)"=w590) -> ()  [unwired: 2 in, 2 out]
      }
      event "Z Move Set": Mouse Down {
        n430 = event-data() -> ()  [unwired: 1 in, 7 out]
        n431 = property on="Z Step SP" class="DigNum (strict)"() -> ("Maximum"=w602:dbl)  [unwired: 2 in, 2 out]
        n432 = property on="Z Step SP" class="DigNum (strict)"() -> ("Minimum"=w601:dbl)  [unwired: 2 in, 2 out]
        n433 = property on="Z steps/rev" class="DigNum (strict)"() -> ("Value"=w608:u32)  [unwired: 2 in, 2 out]
        n434 = property on="Z offset mm" class="DigNum (strict)"() -> ("Value"=w606:dbl)  [unwired: 2 in, 2 out]
        n435 = property on="Z Velocity SP step/sec" class="DigNum (strict)"() -> ("Maximum"=w595:dbl)  [unwired: 2 in, 2 out]
        n436 = property on="Z Velocity SP step/sec" class="DigNum (strict)"() -> ("Minimum"=w594:dbl)  [unwired: 2 in, 2 out]
        n437 = property on="Z Position SP mm" class="DigNum (strict)"() -> ("Value"=w605:dbl)  [unwired: 2 in, 2 out]
        n438 = property on="Z mm/rev" class="DigNum (strict)"() -> ("Value"=w611:dbl)  [unwired: 2 in, 2 out]
        n439 = property on="Z Velocity SP mm/sec" class="DigNum (strict)"() -> ("Value"=w599:dbl)  [unwired: 2 in, 2 out]
        n440 = Subtract(x=w605, y=w606) -> (x-y=w609:dbl)
        n441 = Divide(x=w599, y=w611) -> (x/y=w600:dbl)
        n442 = To Double Precision Float(number=w608) -> (double precision float=w612:dbl)
        n443 = Divide(x=w609, y=w611) -> (x/y=w610:dbl)
        n444 = Multiply(x=w600, y=w612) -> (x*y=w597:dbl)
        n445 = Multiply(x=w610, y=w612) -> (x*y=w604:dbl)
        n446 = In Range and Coerce(upper limit=w595, x=w597, lower limit=w594) -> (coerced(x)=w596:dbl)  [unwired: 1 out]
        n447 = To Long Integer(number=w596) -> (32bit integer=w598:i32)
        n448 = In Range and Coerce(upper limit=w602, x=w604, lower limit=w601) -> (coerced(x)=w603:dbl)  [unwired: 1 out]
        n449 = To Long Integer(number=w603) -> (32bit integer=w607:i32)
        n450 = property on="Z Velocity SP step/sec" class="DigNum (strict)"("Val(Sgnl)"=w598) -> ()  [unwired: 2 in, 2 out]
        n451 = property on="Z Step SP" class="DigNum (strict)"("Val(Sgnl)"=w607) -> ()  [unwired: 2 in, 2 out]
      }
      event "R Move Set": Mouse Down {
        n452 = event-data() -> ()  [unwired: 1 in, 7 out]
        n453 = property on="R Step SP" class="DigNum (strict)"() -> ("Maximum"=w624:dbl)  [unwired: 2 in, 2 out]
        n454 = property on="R Step SP" class="DigNum (strict)"() -> ("Minimum"=w623:dbl)  [unwired: 2 in, 2 out]
        n455 = property on="R steps/rev" class="DigNum (strict)"() -> ("Value"=w630:u32)  [unwired: 2 in, 2 out]
        n456 = property on="R offset deg" class="DigNum (strict)"() -> ("Value"=w628:dbl)  [unwired: 2 in, 2 out]
        n457 = property on="R Velocity SP step/sec" class="DigNum (strict)"() -> ("Maximum"=w617:dbl)  [unwired: 2 in, 2 out]
        n458 = property on="R Velocity SP step/sec" class="DigNum (strict)"() -> ("Minimum"=w616:dbl)  [unwired: 2 in, 2 out]
        n459 = To Double Precision Float(number=w630) -> (double precision float=w615:dbl)
        n460 = property on="SSE:OmniaxR.SV" class="DigNum (strict)"() -> ("Value"=w627:dbl)  [unwired: 2 in, 2 out]
        n461 = property on="R deg/rev" class="DigNum (strict)"() -> ("Value"=w614:dbl)  [unwired: 2 in, 2 out]
        n462 = property on="R Velocity SP deg/sec" class="DigNum (strict)"() -> ("Value"=w621:dbl)  [unwired: 2 in, 2 out]
        n463 = Subtract(x=w627, y=w628) -> (x-y=w631:dbl)
        n464 = Divide(x=w621, y=w614) -> (x/y=w622:dbl)
        n465 = Divide(x=w631, y=w614) -> (x/y=w632:dbl)
        n466 = Multiply(x=w622, y=w615) -> (x*y=w619:dbl)
        n467 = Multiply(x=w632, y=w615) -> (x*y=w626:dbl)
        n468 = Absolute Value(x=w619) -> (abs(x)=w613:dbl)
        n469 = In Range and Coerce(upper limit=w624, x=w626, lower limit=w623) -> (coerced(x)=w625:dbl)  [unwired: 1 out]
        n470 = In Range and Coerce(upper limit=w617, x=w613, lower limit=w616) -> (coerced(x)=w618:dbl)  [unwired: 1 out]
        n471 = To Long Integer(number=w625) -> (32bit integer=w629:i32)
        n472 = To Long Integer(number=w618) -> (32bit integer=w620:i32)
        n473 = property on="R Step SP" class="DigNum (strict)"("Val(Sgnl)"=w629) -> ()  [unwired: 2 in, 2 out]
        n474 = property on="R Velocity SP step/sec" class="DigNum (strict)"("Val(Sgnl)"=w620) -> ()  [unwired: 2 in, 2 out]
      }
      event "Y Scan set": Mouse Down {
        n475 = event-data() -> ()  [unwired: 1 in, 7 out]
        n476 = property on="Y Step SP" class="DigNum (strict)"() -> ("Maximum"=w642:dbl)  [unwired: 2 in, 2 out]
        n477 = property on="Y Step SP" class="DigNum (strict)"() -> ("Minimum"=w643:dbl)  [unwired: 2 in, 2 out]
        n478 = property on="Y steps/rev" class="DigNum (strict)"() -> ("Value"=w648:u32)  [unwired: 2 in, 2 out]
        n479 = To Double Precision Float(number=w648) -> (double precision float=w634:dbl)
        n480 = property on="Y Scan Length SP mm" class="DigNum (strict)"() -> ("Value"=w646:dbl)  [unwired: 2 in, 2 out]
        n481 = property on="Y mm/rev" class="DigNum (strict)"() -> ("Value"=w633:dbl)  [unwired: 2 in, 2 out]
        n482 = property on="Y Scan Velocity SP steps/sec" class="DigNum (strict)"() -> ("Maximum"=w636:dbl)  [unwired: 2 in, 2 out]
        n483 = property on="Y Scan Velocity SP steps/sec" class="DigNum (strict)"() -> ("Minimum"=w635:dbl)  [unwired: 2 in, 2 out]
        n484 = property on="Y Scan Velocity SP mm/sec" class="DigNum (strict)"() -> ("Value"=w640:dbl)  [unwired: 2 in, 2 out]
        n485 = Divide(x=w646, y=w633) -> (x/y=w649:dbl)
        n486 = Multiply(x=w649, y=w634) -> (x*y=w645:dbl)
        n487 = Divide(x=w640, y=w633) -> (x/y=w641:dbl)
        n488 = Multiply(x=w641, y=w634) -> (x*y=w638:dbl)
        n489 = In Range and Coerce(upper limit=w642, x=w645, lower limit=w643) -> (coerced(x)=w644:dbl)  [unwired: 1 out]
        n490 = To Long Integer(number=w644) -> (32bit integer=w647:i32)
        n491 = In Range and Coerce(upper limit=w636, x=w638, lower limit=w635) -> (coerced(x)=w637:dbl)  [unwired: 1 out]
        n492 = To Long Integer(number=w637) -> (32bit integer=w639:i32)
        n493 = property on="Y Scan Length SP steps" class="DigNum (strict)"("Val(Sgnl)"=w647) -> ()  [unwired: 2 in, 2 out]
        n494 = property on="Y Scan Velocity SP steps/sec" class="DigNum (strict)"("Val(Sgnl)"=w639) -> ()  [unwired: 2 in, 2 out]
      }
      event "X Scan set": Mouse Down {
        n495 = event-data() -> ()  [unwired: 1 in, 7 out]
        n496 = property on="X Step SP" class="DigNum (strict)"() -> ("Maximum"=w659:dbl)  [unwired: 2 in, 2 out]
        n497 = property on="X Step SP" class="DigNum (strict)"() -> ("Minimum"=w660:dbl)  [unwired: 2 in, 2 out]
        n498 = property on="X steps/rev" class="DigNum (strict)"() -> ("Value"=w665:u32)  [unwired: 2 in, 2 out]
        n499 = To Double Precision Float(number=w665) -> (double precision float=w651:dbl)
        n500 = property on="X Scan Length SP mm" class="DigNum (strict)"() -> ("Value"=w663:dbl)  [unwired: 2 in, 2 out]
        n501 = property on="X mm/rev" class="DigNum (strict)"() -> ("Value"=w650:dbl)  [unwired: 2 in, 2 out]
        n502 = property on="X Scan Velocity SP steps/sec" class="DigNum (strict)"() -> ("Maximum"=w653:dbl)  [unwired: 2 in, 2 out]
        n503 = property on="X Scan Velocity SP steps/sec" class="DigNum (strict)"() -> ("Minimum"=w652:dbl)  [unwired: 2 in, 2 out]
        n504 = property on="X Scan Velocity SP mm/sec" class="DigNum (strict)"() -> ("Value"=w657:dbl)  [unwired: 2 in, 2 out]
        n505 = Divide(x=w663, y=w650) -> (x/y=w666:dbl)
        n506 = Multiply(x=w666, y=w651) -> (x*y=w662:dbl)
        n507 = Divide(x=w657, y=w650) -> (x/y=w658:dbl)
        n508 = Multiply(x=w658, y=w651) -> (x*y=w655:dbl)
        n509 = In Range and Coerce(upper limit=w659, x=w662, lower limit=w660) -> (coerced(x)=w661:dbl)  [unwired: 1 out]
        n510 = To Long Integer(number=w661) -> (32bit integer=w664:i32)
        n511 = In Range and Coerce(upper limit=w653, x=w655, lower limit=w652) -> (coerced(x)=w654:dbl)  [unwired: 1 out]
        n512 = To Long Integer(number=w654) -> (32bit integer=w656:i32)
        n513 = property on="X Scan Length SP steps" class="DigNum (strict)"("Val(Sgnl)"=w664) -> ()  [unwired: 2 in, 2 out]
        n514 = property on="X Scan Velocity SP steps/sec" class="DigNum (strict)"("Val(Sgnl)"=w656) -> ()  [unwired: 2 in, 2 out]
      }
      event "Z Scan set": Mouse Down {
        n515 = event-data() -> ()  [unwired: 1 in, 7 out]
        n516 = property on="Z Step SP" class="DigNum (strict)"() -> ("Maximum"=w676:dbl)  [unwired: 2 in, 2 out]
        n517 = property on="Z Step SP" class="DigNum (strict)"() -> ("Minimum"=w677:dbl)  [unwired: 2 in, 2 out]
        n518 = property on="Z steps/rev" class="DigNum (strict)"() -> ("Value"=w682:u32)  [unwired: 2 in, 2 out]
        n519 = To Double Precision Float(number=w682) -> (double precision float=w668:dbl)
        n520 = property on="Z Scan Length SP mm" class="DigNum (strict)"() -> ("Value"=w680:dbl)  [unwired: 2 in, 2 out]
        n521 = property on="Z mm/rev" class="DigNum (strict)"() -> ("Value"=w667:dbl)  [unwired: 2 in, 2 out]
        n522 = property on="Z Scan Velocity SP steps/sec" class="DigNum (strict)"() -> ("Maximum"=w670:dbl)  [unwired: 2 in, 2 out]
        n523 = property on="Z Scan Velocity SP steps/sec" class="DigNum (strict)"() -> ("Minimum"=w669:dbl)  [unwired: 2 in, 2 out]
        n524 = property on="Z Scan Velocity SP mm/sec" class="DigNum (strict)"() -> ("Value"=w674:dbl)  [unwired: 2 in, 2 out]
        n525 = Divide(x=w680, y=w667) -> (x/y=w683:dbl)
        n526 = Multiply(x=w683, y=w668) -> (x*y=w679:dbl)
        n527 = Divide(x=w674, y=w667) -> (x/y=w675:dbl)
        n528 = Multiply(x=w675, y=w668) -> (x*y=w672:dbl)
        n529 = In Range and Coerce(upper limit=w676, x=w679, lower limit=w677) -> (coerced(x)=w678:dbl)  [unwired: 1 out]
        n530 = To Long Integer(number=w678) -> (32bit integer=w681:i32)
        n531 = In Range and Coerce(upper limit=w670, x=w672, lower limit=w669) -> (coerced(x)=w671:dbl)  [unwired: 1 out]
        n532 = To Long Integer(number=w671) -> (32bit integer=w673:i32)
        n533 = property on="Z Scan Length SP steps" class="DigNum (strict)"("Val(Sgnl)"=w681) -> ()  [unwired: 2 in, 2 out]
        n534 = property on="Z Scan Velocity SP steps/sec" class="DigNum (strict)"("Val(Sgnl)"=w673) -> ()  [unwired: 2 in, 2 out]
      }
      event "R Scan set": Mouse Down {
        n535 = event-data() -> ()  [unwired: 1 in, 7 out]
        n536 = property on="R Step SP" class="DigNum (strict)"() -> ("Maximum"=w694:dbl)  [unwired: 2 in, 2 out]
        n537 = property on="R Step SP" class="DigNum (strict)"() -> ("Minimum"=w695:dbl)  [unwired: 2 in, 2 out]
        n538 = property on="R steps/rev" class="DigNum (strict)"() -> ("Value"=w700:u32)  [unwired: 2 in, 2 out]
        n539 = property on="R Velocity SP step/sec" class="DigNum (strict)"() -> ("Maximum"=w688:dbl)  [unwired: 2 in, 2 out]
        n540 = To Double Precision Float(number=w700) -> (double precision float=w686:dbl)
        n541 = property on="R Scan Length SP deg" class="DigNum (strict)"() -> ("Value"=w698:dbl)  [unwired: 2 in, 2 out]
        n542 = property on="R deg/rev" class="DigNum (strict)"() -> ("Value"=w685:dbl)  [unwired: 2 in, 2 out]
        n543 = property on="R Scan Velocity SP steps/sec" class="DigNum (strict)"() -> ("Minimum"=w687:dbl)  [unwired: 2 in, 2 out]
        n544 = property on="R Scan Velocity SP deg/sec" class="DigNum (strict)"() -> ("Value"=w692:dbl)  [unwired: 2 in, 2 out]
        n545 = Divide(x=w698, y=w685) -> (x/y=w701:dbl)
        n546 = Multiply(x=w701, y=w686) -> (x*y=w697:dbl)
        n547 = Divide(x=w692, y=w685) -> (x/y=w693:dbl)
        n548 = Multiply(x=w693, y=w686) -> (x*y=w690:dbl)
        n549 = In Range and Coerce(upper limit=w694, x=w697, lower limit=w695) -> (coerced(x)=w696:dbl)  [unwired: 1 out]
        n550 = To Long Integer(number=w696) -> (32bit integer=w699:i32)
        n551 = Absolute Value(x=w690) -> (abs(x)=w684:dbl)
        n552 = property on="R Scan Length SP steps" class="DigNum (strict)"("Val(Sgnl)"=w699) -> ()  [unwired: 2 in, 2 out]
        n553 = In Range and Coerce(upper limit=w688, x=w684, lower limit=w687) -> (coerced(x)=w689:dbl)  [unwired: 1 out]
        n554 = To Long Integer(number=w689) -> (32bit integer=w691:i32)
        n555 = property on="R Scan Velocity SP steps/sec" class="DigNum (strict)"("Val(Sgnl)"=w691) -> ()  [unwired: 2 in, 2 out]
      }
      event "Y Go": Mouse Up {
        n556 = event-data() -> ()  [unwired: 1 in, 7 out]
        n557 = flat-sequence {
          tunnel: [w720] -> w703
          tunnel: [w719] -> w702
          tunnel: [w727] -> w705
          tunnel: [w726] -> w704
          tunnel: w703 -> [w725]
          tunnel: w702 -> [w724]
          tunnel: [w733] -> w706
          tunnel: [w734] -> w707
          tunnel: w705 -> [w734]
          tunnel: w704 -> [w732]
          frame #0 {
            n558 = property on="Scan Go" class="Bool"("DisabledEnum"=T2."Disabled and Grayed Out" ("Disabled")) -> ()  [unwired: 2 in, 2 out]
            n559 = property on="Y Go" class="Bool"("DisabledEnum"=T2."Disabled and Grayed Out" ("Disabled")) -> ()  [unwired: 2 in, 2 out]
          }
          frame #1 {
            n560 = property on="Y Step SP" class="DigNum (strict)"() -> ("Value"=w718:i32)  [unwired: 2 in, 2 out]
            n561 = property on="Y Step PV" class="DigNum (strict)"() -> ("Value"=w717:i32)  [unwired: 2 in, 2 out]
            n562 = property on="Y Backlash" class="DigNum (strict)"() -> ("Value"=w710:i32)  [unwired: 2 in, 2 out]
            n563 = Subtract(x=w718, y=w717) -> (x-y=w716:i32)
            n564 = Sign(1:w710) -> (0:w714:i32)
            n565 = Sign(1:w716) -> (0:w715:i32)
            n566 = Multiply(x=w715, y=w714) -> (x*y=w713:i32)
            n567 = Equal?(x=w713, y=1) -> (x = y?=w711:bool)
            n568 = case shown="False" w711 {
              frame False {
                (unwired) FALSE ("Value (Signaling)")
              }
              frame True {
                (unwired) TRUE ("Value (Signaling)")
              }
            }
          }
          frame #2 {
            # "Velocity Setting"
            n569 = property on="Y Velocity SP step/sec" class="DigNum (strict)"() -> ("Value"=w721:i32)  [unwired: 2 in, 2 out]
            n570 = Number To Decimal String(number=w721) -> (decimal integer string=w722:string)  [unwired: 1 in]
            n571 = call "mDrive Send Command.vi"("Extra"=w722, "Command"=T1."Max Velocity") -> ("error out"=w719:errorcluster, "VISA resource name out"=w720:refnum<visa-resource-name>)  [unwired: 5 in, 1 out]
          }
          frame #3 {
            # "Move to Abs Position"
            n572 = property on="Y Step SP" class="DigNum (strict)"() -> ("Value"=w730:i32)  [unwired: 2 in, 2 out]
            n573 = Number To Decimal String(number=w730) -> (decimal integer string=w729:string)  [unwired: 1 in]
            n574 = call "mDrive Send Command.vi"("error in (no error)"=w724, "Extra"=w729, "Command"=T1."Move to Absolute Position", "VISA resource name"=w725) -> ("error out"=w726:errorcluster, "VISA resource name out"=w727:refnum<visa-resource-name>)  [unwired: 3 in, 1 out]
          }
          frame #4 {
            n575 = call "Time Delay"("error in (no error)"=w732, "Delay Time (s)"=0.1) -> ("error out"=w733:errorcluster)  [unwired: 9 in]
          }
        }
      }
      event "Z Go": Mouse Up {
        n576 = event-data() -> ()  [unwired: 1 in, 7 out]
        n577 = flat-sequence {
          tunnel: [w753] -> w738
          tunnel: [w752] -> w737
          tunnel: [w760] -> w740
          tunnel: [w759] -> w739
          tunnel: w738 -> [w758]
          tunnel: w737 -> [w757]
          tunnel: [w766] -> w736
          tunnel: [w767] -> w735
          tunnel: w740 -> [w767]
          tunnel: w739 -> [w765]
          frame #0 {
            n578 = property on="Scan Go" class="Bool"("DisabledEnum"=T2."Disabled and Grayed Out" ("Disabled")) -> ()  [unwired: 2 in, 2 out]
            n579 = property on="Z Go" class="Bool"("DisabledEnum"=T2."Disabled and Grayed Out" ("Disabled")) -> ()  [unwired: 2 in, 2 out]
          }
          frame #1 {
            n580 = property on="Z Step SP" class="DigNum (strict)"() -> ("Value"=w751:i32)  [unwired: 2 in, 2 out]
            n581 = property on="Z Step PV" class="DigNum (strict)"() -> ("Value"=w750:i32)  [unwired: 2 in, 2 out]
            n582 = property on="Z Backlash" class="DigNum (strict)"() -> ("Value"=w743:i32)  [unwired: 2 in, 2 out]
            n583 = Subtract(x=w751, y=w750) -> (x-y=w749:i32)
            n584 = Sign(1:w743) -> (0:w747:i32)
            n585 = Sign(1:w749) -> (0:w748:i32)
            n586 = Multiply(x=w748, y=w747) -> (x*y=w746:i32)
            n587 = Equal?(x=w746, y=1) -> (x = y?=w744:bool)
            n588 = case shown="True" w744 {
              frame False {
                (unwired) FALSE ("Value (Signaling)")
              }
              frame True {
                (unwired) TRUE ("Value (Signaling)")
              }
            }
          }
          frame #2 {
            # "Velocity Setting"
            n589 = property on="Z Velocity SP step/sec" class="DigNum (strict)"() -> ("Value"=w754:i32)  [unwired: 2 in, 2 out]
            n590 = Number To Decimal String(number=w754) -> (decimal integer string=w755:string)  [unwired: 1 in]
            n591 = call "mDrive Send Command.vi"("Extra"=w755, "Command"=T1."Max Velocity") -> ("error out"=w752:errorcluster, "VISA resource name out"=w753:refnum<visa-resource-name>)  [unwired: 5 in, 1 out]
          }
          frame #3 {
            # "Move to Abs Position"
            n592 = property on="Z Step SP" class="DigNum (strict)"() -> ("Value"=w763:i32)  [unwired: 2 in, 2 out]
            n593 = Number To Decimal String(number=w763) -> (decimal integer string=w762:string)  [unwired: 1 in]
            n594 = call "mDrive Send Command.vi"("error in (no error)"=w757, "Extra"=w762, "Command"=T1."Move to Absolute Position", "VISA resource name"=w758) -> ("error out"=w759:errorcluster, "VISA resource name out"=w760:refnum<visa-resource-name>)  [unwired: 3 in, 1 out]
          }
          frame #4 {
            n595 = call "Time Delay28"("error in (no error)"=w765, "Delay Time (s)"=0.1) -> ("error out"=w766:errorcluster)  [unwired: 9 in]
          }
        }
      }
      event "R Go": Mouse Up {
        n596 = event-data() -> ()  [unwired: 1 in, 7 out]
        n597 = flat-sequence {
          tunnel: w770 -> [w782]
          tunnel: w771 -> [w783]
          tunnel: [w783] -> w773
          tunnel: [w782] -> w772
          tunnel: [w786] -> w775
          tunnel: [w785] -> w774
          tunnel: w773 -> [w788]
          tunnel: w772 -> [w787]
          tunnel: [w806] -> w777
          tunnel: [w805] -> w776
          tunnel: w775 -> [w804]
          tunnel: w774 -> [w803]
          tunnel: [w813] -> w779
          tunnel: [w812] -> w778
          tunnel: w777 -> [w811]
          tunnel: w776 -> [w810]
          tunnel: [w819] -> w769
          tunnel: [w820] -> w768
          tunnel: w779 -> [w820]
          tunnel: w778 -> [w818]
          frame #0 {
            n598 = property on="Scan Go" class="Bool"("DisabledEnum"=T2."Disabled and Grayed Out" ("Disabled")) -> ()  [unwired: 2 in, 2 out]
            n599 = property on="R Go" class="Bool"("DisabledEnum"=T2."Disabled and Grayed Out" ("Disabled")) -> ()  [unwired: 2 in, 2 out]
          }
          frame #1 {
            n600 = property on="R Step SP" class="DigNum (strict)"() -> ("Value"=w796:i32)  [unwired: 2 in, 2 out]
            n601 = property on="R Step PV" class="DigNum (strict)"() -> ("Value"=w795:i32)  [unwired: 2 in, 2 out]
            n602 = property on="R Backlash" class="DigNum (strict)"() -> ("Value"=w784:i32)  [unwired: 2 in, 2 out]
            n603 = Subtract(x=w796, y=w795) -> (x-y=w794:i32)
            n604 = Sign(1:w784) -> (0:w792:i32)
            n605 = Sign(1:w794) -> (0:w793:i32)
            n606 = Multiply(x=w793, y=w792) -> (x*y=w791:i32)
            n607 = Equal?(x=w791, y=1) -> (x = y?=w789:bool)
            n608 = case shown="True" w789 {
              tunnel: w788 -> [w799 w801]
              tunnel: w787 -> [w798 w800]
              tunnel: [w798 w800] -> w786
              tunnel: [w799 w801] -> w785
              frame False {
                n609 = property on="R Backlash corr" class="Bool (strict)"("Val(Sgnl)"=FALSE ("Value (Signaling)")) -> ()  [unwired: 2 in, 2 out]
              }
              frame True {
                n610 = property on="R Backlash corr" class="Bool (strict)"("Val(Sgnl)"=TRUE ("Value (Signaling)")) -> ()  [unwired: 2 in, 2 out]
              }
            }
          }
          frame #2 {
            # "Velocity Setting"
            n611 = property on="R Velocity SP step/sec" class="DigNum (strict)"() -> ("Value"=w807:i32)  [unwired: 2 in, 2 out]
            n612 = Number To Decimal String(number=w807) -> (decimal integer string=w808:string)  [unwired: 1 in]
            n613 = call "mDrive Send Command.vi"("error in (no error)"=w804, "Extra"=w808, "Command"=T1."Max Velocity", "VISA resource name"=w803) -> ("error out"=w805:errorcluster, "VISA resource name out"=w806:refnum<visa-resource-name>)  [unwired: 3 in, 1 out]
          }
          frame #3 {
            # "Move to Abs Position"
            n614 = property on="R Step SP" class="DigNum (strict)"() -> ("Value"=w816:i32)  [unwired: 2 in, 2 out]
            n615 = Number To Decimal String(number=w816) -> (decimal integer string=w815:string)  [unwired: 1 in]
            n616 = call "mDrive Send Command.vi"("error in (no error)"=w810, "Extra"=w815, "Command"=T1."Move to Absolute Position", "VISA resource name"=w811) -> ("error out"=w812:errorcluster, "VISA resource name out"=w813:refnum<visa-resource-name>)  [unwired: 3 in, 1 out]
          }
          frame #4 {
            n617 = call "Time Delay29"("error in (no error)"=w818, "Delay Time (s)"=0.1) -> ("error out"=w819:errorcluster)  [unwired: 9 in]
          }
        }
      }
      event "X Go": Mouse Up {
        n618 = event-data() -> ()  [unwired: 1 in, 7 out]
        n619 = flat-sequence {
          tunnel: [w839] -> w824
          tunnel: [w838] -> w823
          tunnel: [w846] -> w826
          tunnel: [w845] -> w825
          tunnel: w824 -> [w844]
          tunnel: w823 -> [w843]
          tunnel: [w852] -> w821
          tunnel: [w853] -> w822
          tunnel: w826 -> [w853]
          tunnel: w825 -> [w851]
          frame #0 {
            n620 = property on="Scan Go" class="Bool"("DisabledEnum"=T2."Disabled and Grayed Out" ("Disabled")) -> ()  [unwired: 2 in, 2 out]
            n621 = property on="X Go" class="Bool"("DisabledEnum"=T2."Disabled and Grayed Out" ("Disabled")) -> ()  [unwired: 2 in, 2 out]
          }
          frame #1 {
            n622 = property on="X Step SP" class="DigNum (strict)"() -> ("Value"=w837:i32)  [unwired: 2 in, 2 out]
            n623 = property on="X Step PV" class="DigNum (strict)"() -> ("Value"=w836:i32)  [unwired: 2 in, 2 out]
            n624 = property on="X Backlash" class="DigNum (strict)"() -> ("Value"=w829:i32)  [unwired: 2 in, 2 out]
            n625 = Subtract(x=w837, y=w836) -> (x-y=w835:i32)
            n626 = Sign(1:w829) -> (0:w833:i32)
            n627 = Sign(1:w835) -> (0:w834:i32)
            n628 = Multiply(x=w834, y=w833) -> (x*y=w832:i32)
            n629 = Equal?(x=w832, y=1) -> (x = y?=w830:bool)
            n630 = case shown="True" w830 {
              frame False {
                (unwired) FALSE ("Value (Signaling)")
              }
              frame True {
                (unwired) TRUE ("Value (Signaling)")
              }
            }
          }
          frame #2 {
            # "Velocity Setting"
            n631 = property on="X Velocity SP step/sec" class="DigNum (strict)"() -> ("Value"=w840:i32)  [unwired: 2 in, 2 out]
            n632 = Number To Decimal String(number=w840) -> (decimal integer string=w841:string)  [unwired: 1 in]
            n633 = call "mDrive Send Command.vi"("Extra"=w841, "Command"=T1."Max Velocity") -> ("error out"=w838:errorcluster, "VISA resource name out"=w839:refnum<visa-resource-name>)  [unwired: 5 in, 1 out]
          }
          frame #3 {
            # "Move to Abs Position"
            n634 = property on="X Step SP" class="DigNum (strict)"() -> ("Value"=w849:i32)  [unwired: 2 in, 2 out]
            n635 = Number To Decimal String(number=w849) -> (decimal integer string=w848:string)  [unwired: 1 in]
            n636 = call "mDrive Send Command.vi"("error in (no error)"=w843, "Extra"=w848, "Command"=T1."Move to Absolute Position", "VISA resource name"=w844) -> ("error out"=w845:errorcluster, "VISA resource name out"=w846:refnum<visa-resource-name>)  [unwired: 3 in, 1 out]
          }
          frame #4 {
            n637 = call "Time Delay15"("error in (no error)"=w851, "Delay Time (s)"=0.1) -> ("error out"=w852:errorcluster)  [unwired: 9 in]
          }
        }
      }
      event "X Scan OK": Mouse Up {
        n638 = event-data() -> ()  [unwired: 1 in, 7 out]
        n639 = flat-sequence {
          tunnel: [w865] -> w859
          tunnel: [w863] -> w858
          tunnel: w859 -> [w879]
          tunnel: w858 -> [w878]
          tunnel: [w879] -> w855
          tunnel: [w878] -> w854
          tunnel: [w881] -> w856
          tunnel: [w882] -> w857
          tunnel: w855 -> [w882]
          tunnel: w854 -> [w881]
          frame #0 {
            # "VELOCITY"
            n640 = property on="X Scan Velocity SP steps/sec" class="DigNum (strict)"() -> ("Value"=w866:i32)  [unwired: 2 in, 2 out]
            n641 = Number To Decimal String(number=w866) -> (decimal integer string=w867:string)  [unwired: 1 in]
            n642 = call "mDrive Send Command.vi"("Extra"=w867, "Command"=T1."Max Velocity") -> ("error out"=w868:errorcluster, "VISA resource name out"=w873:refnum<visa-resource-name>)  [unwired: 5 in, 1 out]
            n643 = call "Time Delay9"("error in (no error)"=w868) -> ("error out"=w871:errorcluster)  [unwired: 10 in]
            n644 = call "mDrive Send Command.vi"("error in (no error)"=w871, "Extra"="VM", "Command"=T1."Print Parameter", "VISA resource name"=w873) -> ("error out"=w864:errorcluster, "read buffer"=w869:string, "VISA resource name out"=w865:refnum<visa-resource-name>)  [unwired: 3 in]
            n645 = call "Time Delay10"("error in (no error)"=w864) -> ("error out"=w863:errorcluster)  [unwired: 10 in]
            n646 = Decimal String To Number(string=w869, offset=0) -> (number=w872:i32)  [unwired: 1 in, 1 out]
            n647 = property on="X velocity PV step/sec" class="DigNum (strict)"("Val(Sgnl)"=w872) -> ()  [unwired: 2 in, 2 out]
          }
          frame #1 {
            (unwired) TRUE ("Slew Ready 2")
            n648 = property on="Scan Cancel" class="Bool"("DisabledEnum"=T2."Enabled" ("Disabled")) -> ()  [unwired: 2 in, 2 out]
            n649 = property on="Scan Go" class="Bool"("DisabledEnum"=T2."Enabled" ("Disabled")) -> ()  [unwired: 2 in, 2 out]
            n650 = property on="X Scan Length SP steps" class="DigNum (strict)"("DisabledEnum"=T2."Disabled and Grayed Out" ("Disabled")) -> ()  [unwired: 2 in, 2 out]
            n651 = property on="X Scan Velocity SP steps/sec" class="DigNum (strict)"("DisabledEnum"=T2."Disabled and Grayed Out" ("Disabled")) -> ()  [unwired: 2 in, 2 out]
          }
          frame #2 {
            n652 = property on="X Go" class="Bool"("DisabledEnum"=T2."Disabled and Grayed Out" ("Disabled")) -> ()  [unwired: 2 in, 2 out]
          }
        }
      }
      event "Y Scan OK": Mouse Up {
        n653 = event-data() -> ()  [unwired: 1 in, 7 out]
        n654 = flat-sequence {
          tunnel: [w894] -> w887
          tunnel: [w892] -> w886
          tunnel: w887 -> [w908]
          tunnel: w886 -> [w907]
          tunnel: [w908] -> w884
          tunnel: [w907] -> w883
          tunnel: [w910] -> w888
          tunnel: [w911] -> w885
          tunnel: w884 -> [w911]
          tunnel: w883 -> [w910]
          frame #0 {
            # "VELOCITY"
            n655 = property on="Y Scan Velocity SP steps/sec" class="DigNum (strict)"() -> ("Value"=w895:i32)  [unwired: 2 in, 2 out]
            n656 = Number To Decimal String(number=w895) -> (decimal integer string=w896:string)  [unwired: 1 in]
            n657 = call "mDrive Send Command.vi"("Extra"=w896, "Command"=T1."Max Velocity") -> ("error out"=w897:errorcluster, "VISA resource name out"=w902:refnum<visa-resource-name>)  [unwired: 5 in, 1 out]
            n658 = call "Time Delay5"("error in (no error)"=w897) -> ("error out"=w900:errorcluster)  [unwired: 10 in]
            n659 = call "mDrive Send Command.vi"("error in (no error)"=w900, "Extra"="VM", "Command"=T1."Print Parameter", "VISA resource name"=w902) -> ("error out"=w893:errorcluster, "read buffer"=w898:string, "VISA resource name out"=w894:refnum<visa-resource-name>)  [unwired: 3 in]
            n660 = Decimal String To Number(string=w898, offset=0) -> (number=w901:i32)  [unwired: 1 in, 1 out]
            n661 = property on="Y velocity PV step/sec" class="DigNum (strict)"("Val(Sgnl)"=w901) -> ()  [unwired: 2 in, 2 out]
            n662 = call "Time Delay6"("error in (no error)"=w893) -> ("error out"=w892:errorcluster)  [unwired: 10 in]
          }
          frame #1 {
            (unwired) TRUE ("Slew Ready 2")
            n663 = property on="Scan Cancel" class="Bool"("DisabledEnum"=T2."Enabled" ("Disabled")) -> ()  [unwired: 2 in, 2 out]
            n664 = property on="Scan Go" class="Bool"("DisabledEnum"=T2."Enabled" ("Disabled")) -> ()  [unwired: 2 in, 2 out]
            n665 = property on="Y Scan Length SP steps" class="DigNum (strict)"("DisabledEnum"=T2."Disabled and Grayed Out" ("Disabled")) -> ()  [unwired: 2 in, 2 out]
            n666 = property on="Y Scan Velocity SP steps/sec" class="DigNum (strict)"("DisabledEnum"=T2."Disabled and Grayed Out" ("Disabled")) -> ()  [unwired: 2 in, 2 out]
          }
          frame #2 {
            n667 = property on="Y Go" class="Bool"("DisabledEnum"=T2."Disabled and Grayed Out" ("Disabled")) -> ()  [unwired: 2 in, 2 out]
          }
        }
      }
      event "Z Scan OK": Mouse Up {
        n668 = event-data() -> ()  [unwired: 1 in, 7 out]
        n669 = flat-sequence {
          tunnel: [w923] -> w917
          tunnel: [w921] -> w916
          tunnel: w917 -> [w937]
          tunnel: w916 -> [w936]
          tunnel: [w937] -> w915
          tunnel: [w936] -> w914
          tunnel: [w939] -> w913
          tunnel: [w940] -> w912
          tunnel: w915 -> [w940]
          tunnel: w914 -> [w939]
          frame #0 {
            # "VELOCITY"
            n670 = property on="Z Scan Velocity SP steps/sec" class="DigNum (strict)"() -> ("Value"=w924:i32)  [unwired: 2 in, 2 out]
            n671 = Number To Decimal String(number=w924) -> (decimal integer string=w925:string)  [unwired: 1 in]
            n672 = call "mDrive Send Command.vi"("Extra"=w925, "Command"=T1."Max Velocity") -> ("error out"=w926:errorcluster, "VISA resource name out"=w931:refnum<visa-resource-name>)  [unwired: 5 in, 1 out]
            n673 = call "Time Delay24"("error in (no error)"=w926) -> ("error out"=w929:errorcluster)  [unwired: 10 in]
            n674 = call "mDrive Send Command.vi"("error in (no error)"=w929, "Extra"="VM", "Command"=T1."Print Parameter", "VISA resource name"=w931) -> ("error out"=w922:errorcluster, "read buffer"=w927:string, "VISA resource name out"=w923:refnum<visa-resource-name>)  [unwired: 3 in]
            n675 = Decimal String To Number(string=w927, offset=0) -> (number=w930:i32)  [unwired: 1 in, 1 out]
            n676 = property on="Z  velocity PV step/sec" class="DigNum (strict)"("Val(Sgnl)"=w930) -> ()  [unwired: 2 in, 2 out]
            n677 = call "Time Delay25"("error in (no error)"=w922) -> ("error out"=w921:errorcluster)  [unwired: 10 in]
          }
          frame #1 {
            (unwired) TRUE ("Slew Ready 2")
            n678 = property on="Scan Cancel" class="Bool"("DisabledEnum"=T2."Enabled" ("Disabled")) -> ()  [unwired: 2 in, 2 out]
            n679 = property on="Scan Go" class="Bool"("DisabledEnum"=T2."Enabled" ("Disabled")) -> ()  [unwired: 2 in, 2 out]
            n680 = property on="Z Scan Length SP steps" class="DigNum (strict)"("DisabledEnum"=T2."Disabled and Grayed Out" ("Disabled")) -> ()  [unwired: 2 in, 2 out]
            n681 = property on="Z Scan Velocity SP steps/sec" class="DigNum (strict)"("DisabledEnum"=T2."Disabled and Grayed Out" ("Disabled")) -> ()  [unwired: 2 in, 2 out]
          }
          frame #2 {
            n682 = property on="Z Go" class="Bool"("DisabledEnum"=T2."Disabled and Grayed Out" ("Disabled")) -> ()  [unwired: 2 in, 2 out]
          }
        }
      }
      event "R Scan OK": Mouse Up {
        n683 = event-data() -> ()  [unwired: 1 in, 7 out]
        n684 = flat-sequence {
          tunnel: [w956] -> w948
          tunnel: [w954] -> w947
          tunnel: w944 -> [w950]
          tunnel: w943 -> [w949]
          tunnel: w948 -> [w971]
          tunnel: w947 -> [w970]
          tunnel: [w971] -> w946
          tunnel: [w970] -> w945
          tunnel: [w973] -> w941
          tunnel: [w974] -> w942
          tunnel: w946 -> [w974]
          tunnel: w945 -> [w973]
          frame #0 {
            # "VELOCITY"
            n685 = property on="R Scan Velocity SP steps/sec" class="DigNum (strict)"() -> ("Value"=w957:i32)  [unwired: 2 in, 2 out]
            n686 = Number To Decimal String(number=w957) -> (decimal integer string=w958:string)  [unwired: 1 in]
            n687 = call "mDrive Send Command.vi"("error in (no error)"=w949, "Extra"=w958, "Command"=T1."Max Velocity", "VISA resource name"=w950) -> ("error out"=w959:errorcluster, "VISA resource name out"=w964:refnum<visa-resource-name>)  [unwired: 3 in, 1 out]
            n688 = call "Time Delay26"("error in (no error)"=w959) -> ("error out"=w962:errorcluster)  [unwired: 10 in]
            n689 = call "mDrive Send Command.vi"("error in (no error)"=w962, "Extra"="VM", "Command"=T1."Print Parameter", "VISA resource name"=w964) -> ("error out"=w955:errorcluster, "read buffer"=w960:string, "VISA resource name out"=w956:refnum<visa-resource-name>)  [unwired: 3 in]
            n690 = Decimal String To Number(string=w960, offset=0) -> (number=w963:i32)  [unwired: 1 in, 1 out]
            n691 = property on="R velocity PV step/sec" class="DigNum (strict)"("Val(Sgnl)"=w963) -> ()  [unwired: 2 in, 2 out]
            n692 = call "Time Delay27"("error in (no error)"=w955) -> ("error out"=w954:errorcluster)  [unwired: 10 in]
          }
          frame #1 {
            n693 = property on="R Scan" class="Bool (strict)"("Val(Sgnl)"=TRUE ("Slew Ready 2")) -> ()  [unwired: 2 in, 2 out]
            n694 = property on="Scan Cancel" class="Bool"("DisabledEnum"=T2."Enabled" ("Disabled")) -> ()  [unwired: 2 in, 2 out]
            n695 = property on="Scan Go" class="Bool"("DisabledEnum"=T2."Enabled" ("Disabled")) -> ()  [unwired: 2 in, 2 out]
            n696 = property on="R Scan Length SP steps" class="DigNum (strict)"("DisabledEnum"=T2."Disabled and Grayed Out" ("Disabled")) -> ()  [unwired: 2 in, 2 out]
            n697 = property on="R Scan Velocity SP steps/sec" class="DigNum (strict)"("DisabledEnum"=T2."Disabled and Grayed Out" ("Disabled")) -> ()  [unwired: 2 in, 2 out]
          }
          frame #2 {
            n698 = property on="R Go" class="Bool"("DisabledEnum"=T2."Disabled and Grayed Out" ("Disabled")) -> ()  [unwired: 2 in, 2 out]
          }
        }
      }
      event Application Instance Close? {
        n699 = event-data() -> ()  [unwired: 1 in, 4 out]
        n700 = event-data() -> ()  [unwired: 3 in, 1 out]
      }
      event "Stop": Mouse Down {
        n701 = event-data() -> ()  [unwired: 1 in, 7 out]
        n702 = flat-sequence {
          tunnel: [w994] -> w982
          tunnel: [w993] -> w981
          frame #0 {
            n703 = call "mDrive Send Command.vi"("Command"=T1."Stop") -> ("error out"=w993:errorcluster, "VISA resource name out"=w994:refnum<visa-resource-name>)  [unwired: 6 in, 1 out]
          }
        }
        n704 = flat-sequence {
          tunnel: [w998] -> w984
          tunnel: [w997] -> w983
          frame #0 {
            n705 = call "mDrive Send Command.vi"("Command"=T1."Stop") -> ("error out"=w997:errorcluster, "VISA resource name out"=w998:refnum<visa-resource-name>)  [unwired: 6 in, 1 out]
          }
        }
        n706 = flat-sequence {
          tunnel: [w991] -> w980
          tunnel: [w990] -> w979
          frame #0 {
            n707 = call "mDrive Send Command.vi"("Command"=T1."Stop") -> ("error out"=w990:errorcluster, "VISA resource name out"=w991:refnum<visa-resource-name>)  [unwired: 6 in, 1 out]
          }
        }
        n708 = flat-sequence {
          tunnel: w978 -> [w989]
          tunnel: w977 -> [w988]
          tunnel: [w987] -> w976
          tunnel: [w985] -> _
          tunnel: [w985] -> w975
          frame #0 {
            n709 = call "mDrive Send Command.vi"("error in (no error)"=w988, "Command"=T1."Stop", "VISA resource name"=w989) -> ("error out"=w985:errorcluster, "VISA resource name out"=w987:refnum<visa-resource-name>)  [unwired: 4 in, 1 out]
          }
        }
      }
      event "Scan Cancel": Mouse Down {
        n710 = event-data() -> ()  [unwired: 1 in, 7 out]
        n711 = flat-sequence {
          tunnel: [w1044] -> w1012
          tunnel: [w1043] -> w1011
          tunnel: [w1050] -> w1009
          tunnel: [w1051] -> w1010
          tunnel: w1012 -> [w1051]
          tunnel: w1011 -> [w1050]
          frame #0 {
            n712 = call "mDrive Send Command.vi"("Command"=T1."Stop") -> ("error out"=w1043:errorcluster, "VISA resource name out"=w1044:refnum<visa-resource-name>)  [unwired: 6 in, 1 out]
          }
          frame #1 {
            (unwired) FALSE ("Slew Ready")
            n713 = property on="X Scan set" class="Bool"("DisabledEnum"=T2."Enabled" ("Disabled")) -> ()  [unwired: 2 in, 2 out]
            n714 = property on="X Scan Velocity SP steps/sec" class="DigNum (strict)"("DisabledEnum"=T2."Enabled" ("Disabled")) -> ()  [unwired: 2 in, 2 out]
            n715 = property on="X Scan Length SP steps" class="DigNum (strict)"("DisabledEnum"=T2."Enabled" ("Disabled")) -> ()  [unwired: 2 in, 2 out]
            n716 = property on="X Go" class="Bool"("DisabledEnum"=T2."Enabled" ("Disabled")) -> ()  [unwired: 2 in, 2 out]
            n717 = property on="X Scan OK" class="Bool"("DisabledEnum"=T2."Enabled" ("Disabled")) -> ()  [unwired: 2 in, 2 out]
          }
        }
        n718 = flat-sequence {
          tunnel: [w1054] -> w1014
          tunnel: [w1053] -> w1013
          tunnel: [w1060] -> w1017
          tunnel: [w1061] -> w1018
          tunnel: w1014 -> [w1061]
          tunnel: w1013 -> [w1060]
          frame #0 {
            n719 = call "mDrive Send Command.vi"("Command"=T1."Stop") -> ("error out"=w1053:errorcluster, "VISA resource name out"=w1054:refnum<visa-resource-name>)  [unwired: 6 in, 1 out]
          }
          frame #1 {
            (unwired) FALSE ("Slew Ready")
            n720 = property on="Y Go" class="Bool"("DisabledEnum"=T2."Enabled" ("Disabled")) -> ()  [unwired: 2 in, 2 out]
            n721 = property on="Y Scan Velocity SP steps/sec" class="DigNum (strict)"("DisabledEnum"=T2."Enabled" ("Disabled")) -> ()  [unwired: 2 in, 2 out]
            n722 = property on="Y Scan set" class="Bool"("DisabledEnum"=T2."Enabled" ("Disabled")) -> ()  [unwired: 2 in, 2 out]
            n723 = property on="Y Scan OK" class="Bool"("DisabledEnum"=T2."Enabled" ("Disabled")) -> ()  [unwired: 2 in, 2 out]
            n724 = property on="Y Scan Length SP steps" class="DigNum (strict)"("DisabledEnum"=T2."Enabled" ("Disabled")) -> ()  [unwired: 2 in, 2 out]
          }
        }
        n725 = flat-sequence {
          tunnel: [w1034] -> w1008
          tunnel: [w1033] -> w1007
          tunnel: [w1040] -> w1005
          tunnel: [w1041] -> w1006
          tunnel: w1008 -> [w1041]
          tunnel: w1007 -> [w1040]
          frame #0 {
            n726 = call "mDrive Send Command.vi"("Command"=T1."Stop") -> ("error out"=w1033:errorcluster, "VISA resource name out"=w1034:refnum<visa-resource-name>)  [unwired: 6 in, 1 out]
          }
          frame #1 {
            (unwired) FALSE ("Slew Ready")
            n727 = property on="Z Scan set" class="Bool"("DisabledEnum"=T2."Enabled" ("Disabled")) -> ()  [unwired: 2 in, 2 out]
            n728 = property on="Z Scan Velocity SP steps/sec" class="DigNum (strict)"("DisabledEnum"=T2."Enabled" ("Disabled")) -> ()  [unwired: 2 in, 2 out]
            n729 = property on="Z Scan Length SP steps" class="DigNum (strict)"("DisabledEnum"=T2."Enabled" ("Disabled")) -> ()  [unwired: 2 in, 2 out]
            n730 = property on="Z Go" class="Bool"("DisabledEnum"=T2."Enabled" ("Disabled")) -> ()  [unwired: 2 in, 2 out]
            n731 = property on="Z Scan OK" class="Bool"("DisabledEnum"=T2."Enabled" ("Disabled")) -> ()  [unwired: 2 in, 2 out]
          }
        }
        n732 = flat-sequence {
          tunnel: [w1023] -> w1004
          tunnel: [w1022] -> w1003
          tunnel: w1002 -> [w1020]
          tunnel: w1001 -> [w1019]
          tunnel: [w1030] -> w999
          tunnel: [w1031] -> w1000
          tunnel: w1004 -> [w1031]
          tunnel: w1003 -> [w1030]
          frame #0 {
            n733 = call "mDrive Send Command.vi"("error in (no error)"=w1019, "Command"=T1."Stop", "VISA resource name"=w1020) -> ("error out"=w1022:errorcluster, "VISA resource name out"=w1023:refnum<visa-resource-name>)  [unwired: 4 in, 1 out]
          }
          frame #1 {
            n734 = property on="R Scan" class="Bool (strict)"("Value"=FALSE ("Slew Ready")) -> ()  [unwired: 2 in, 2 out]
            n735 = property on="R Scan Velocity SP steps/sec" class="DigNum (strict)"("DisabledEnum"=T2."Enabled" ("Disabled")) -> ()  [unwired: 2 in, 2 out]
            n736 = property on="R Go" class="Bool"("DisabledEnum"=T2."Enabled" ("Disabled")) -> ()  [unwired: 2 in, 2 out]
            n737 = property on="R Scan OK" class="Bool"("DisabledEnum"=T2."Enabled" ("Disabled")) -> ()  [unwired: 2 in, 2 out]
            n738 = property on="R Scan Length SP steps" class="DigNum (strict)"("DisabledEnum"=T2."Enabled" ("Disabled")) -> ()  [unwired: 2 in, 2 out]
            n739 = property on="R Scan set" class="Bool"("DisabledEnum"=T2."Enabled" ("Disabled")) -> ()  [unwired: 2 in, 2 out]
          }
        }
        n740 = property on="Scan Go" class="Bool"("DisabledEnum"=T2."Disabled and Grayed Out" ("Disabled")) -> ()  [unwired: 2 in, 2 out]
        n741 = property on="Scan Cancel" class="Bool"("DisabledEnum"=T2."Disabled and Grayed Out" ("Disabled")) -> ()  [unwired: 2 in, 2 out]
      }
      event "Scan Go": Mouse Up {
        n742 = event-data() -> ()  [unwired: 1 in, 7 out]
        n743 = flat-sequence {
          tunnel: [w1081] -> w1077
          tunnel: [w1080] -> w1076
          tunnel: [w1079] -> w1069
          tunnel: w1068 -> [w1079]
          tunnel: [w1078] -> w1067
          tunnel: w1066 -> [w1078]
          tunnel: w1077 -> [w1093]
          tunnel: w1076 -> [w1094]
          tunnel: [w1093] -> w1074
          tunnel: [w1092] -> w1072
          tunnel: [w1091] -> w1070
          tunnel: w1069 -> [w1090]
          tunnel: w1067 -> [w1089]
          tunnel: [w1104] -> w1075
          tunnel: w1074 -> [w1104]
          tunnel: [w1103] -> w1073
          tunnel: w1072 -> [w1103]
          tunnel: [w1102] -> w1071
          tunnel: w1070 -> [w1102]
          tunnel: w1075 -> [w1110]
          tunnel: w1073 -> [w1109]
          tunnel: w1071 -> [w1108]
          tunnel: [w1107] -> w1065
          tunnel: [w1106] -> w1062
          tunnel: w1065 -> [w1121]
          tunnel: [w1121] -> w1064
          tunnel: [w1120] -> w1063
          tunnel: w1062 -> [w1120]
          frame #0 {
            n744 = property on="R Scan" class="Bool (strict)"() -> ("Value"=w1081:bool)  [unwired: 2 in, 2 out]
            n745 = case shown="True" w1081 {
              tunnel: ["" w1083] -> w1080
              frame False {
              }
              frame True {
                n746 = property on="R Scan Length SP steps" class="DigNum (strict)"() -> ("Value"=w1088:i32)  [unwired: 2 in, 2 out]
                n747 = Number To Decimal String(number=w1088) -> (decimal integer string=w1085:string)  [unwired: 1 in]
                n748 = call <vilib>:"Space Constant.vi"() -> ("String"=w1086:string)
                n749 = Concatenate Strings("MR", w1086, w1085, "\r") -> (w1083:string)
              }
            }
          }
          frame #1 {
            n750 = case shown="True" w1093 {
              tunnel: [w1096 w1101] -> w1092
              tunnel: [w1095 w1100] -> w1091
              tunnel: w1094 -> [_ w1099]
              tunnel: w1090 -> [w1096 w1098]
              tunnel: w1089 -> [w1095 w1097]
              frame False {
              }
              frame True {
                n751 = VISA Write(VISA resource name=w1098, write buffer=w1099, error in (no error)=w1097) -> (VISA resource name out=w1101:refnum<visa-resource-name>, error out=w1100:errorcluster)  [unwired: 1 out]
              }
            }
          }
          frame #2 {
            n752 = call "Time Delay7"("Delay Time (s)"=0.1) -> ()  [unwired: 10 in, 1 out]
          }
          frame #3 {
            n753 = case shown="True" w1110 {
              tunnel: w1109 -> [w1112 w1116]
              tunnel: w1108 -> [w1111 w1115]
              tunnel: [w1112 w1114] -> w1107
              tunnel: [w1111 w1113] -> w1106
              frame False {
              }
              frame True {
                n754 = property class="Instr"(reference=w1116, error in=w1115) -> (reference out=w1118:refnum<visa-resource-name>, error out=w1117:errorcluster, "Serial Settings:Number of Bytes at Serial Port"=w1119:u32)
                n755 = VISA Read(VISA resource name=w1118, byte count=w1119, error in (no error)=w1117) -> (VISA resource name out=w1114:refnum<visa-resource-name>, error out=w1113:errorcluster)  [unwired: 2 out]
              }
            }
          }
          frame #4 {
            (unwired) FALSE ("Slew Ready 2")
            (unwired) FALSE ("Slew Ready 2")
            (unwired) FALSE ("Slew Ready 2")
            n756 = property on="R Scan" class="Bool (strict)"("Val(Sgnl)"=FALSE ("Slew Ready 2")) -> ()  [unwired: 2 in, 2 out]
            n757 = property on="Z Scan Velocity SP steps/sec" class="DigNum (strict)"("DisabledEnum"=T2."Enabled" ("Disabled")) -> ()  [unwired: 2 in, 2 out]
            n758 = property on="X Scan Length SP steps" class="DigNum (strict)"("DisabledEnum"=T2."Enabled" ("Disabled")) -> ()  [unwired: 2 in, 2 out]
            n759 = property on="Y Scan Selocity SP steps/sec" class="DigNum (strict)"("DisabledEnum"=T2."Enabled" ("Disabled")) -> ()  [unwired: 2 in, 2 out]
            n760 = property on="Z Scan Length SP steps" class="DigNum (strict)"("DisabledEnum"=T2."Enabled" ("Disabled")) -> ()  [unwired: 2 in, 2 out]
            n761 = property on="Y Scan Length SP steps" class="DigNum (strict)"("DisabledEnum"=T2."Enabled" ("Disabled")) -> ()  [unwired: 2 in, 2 out]
            n762 = property on="X Scan Velocity SP steps/sec" class="DigNum (strict)"("DisabledEnum"=T2."Enabled" ("Disabled")) -> ()  [unwired: 2 in, 2 out]
            n763 = property on="R Scan Velocity SP steps/sec" class="DigNum (strict)"("DisabledEnum"=T2."Enabled" ("Disabled")) -> ()  [unwired: 2 in, 2 out]
            n764 = property on="R Scan Length SP steps" class="DigNum (strict)"("DisabledEnum"=T2."Enabled" ("Disabled")) -> ()  [unwired: 2 in, 2 out]
            n765 = property on="Scan Go" class="Bool"("DisabledEnum"=T2."Disabled and Grayed Out" ("Disabled")) -> ()  [unwired: 2 in, 2 out]
            n766 = property on="Scan Cancel" class="Bool"("DisabledEnum"=T2."Disabled and Grayed Out" ("Disabled")) -> ()  [unwired: 2 in, 2 out]
          }
        }
      }
      event "Reset": Mouse Down {
        n767 = event-data() -> ()  [unwired: 1 in, 7 out]
        n768 = flat-sequence {
          tunnel: [w1138] -> w1134
          tunnel: [w1140] -> w1133
          tunnel: w1136 -> [w1139]
          tunnel: w1135 -> [w1137]
          frame #0 {
            n769 = property on="Reset R Motor Steps" class="DigNum (strict)"() -> ("Value"=w1141:i32)  [unwired: 2 in, 2 out]
            n770 = Number To Decimal String(number=w1141) -> (decimal integer string=w1142:string)  [unwired: 1 in]
            n771 = call "mDrive Send Command.vi"("error in (no error)"=w1137, "Extra"=w1142, "Command"=T1."Set Current Position", "VISA resource name"=w1139) -> ("error out"=w1140:errorcluster, "VISA resource name out"=w1138:refnum<visa-resource-name>)  [unwired: 3 in, 1 out]
          }
        }
      }
    }
    n772 = case shown="True" "Set Button" {
      tunnel: "Preset positions" -> [_ w234]
      frame False {
      }
      frame True {
        n773 = property on="Presets" class="Arr (strict)"() -> ("Value"=w231:i32[][])  [unwired: 2 in, 2 out]
        n774 = Index Array(array=w231, index (row)=w234) -> (element=w233:i32[])  [unwired: 1 in]
        n775 = Array To Cluster(array=w233) -> (cluster=w232:T5)
        n776 = Unbundle(w232) -> ("Value[0]"=w230:i32, "Value[1]"=w229:i32, "Value[2]"=w228:i32, "Value[3]"=w227:i32)  [unwired: 5 out]
        n777 = property on="X Step SP" class="DigNum (strict)"("Val(Sgnl)"=w230) -> ()  [unwired: 2 in, 2 out]
        n778 = property on="Y Step SP" class="DigNum (strict)"("Val(Sgnl)"=w229) -> ()  [unwired: 2 in, 2 out]
        n779 = property on="Z Step SP" class="DigNum (strict)"("Val(Sgnl)"=w228) -> ()  [unwired: 2 in, 2 out]
        n780 = property on="R Step SP" class="DigNum (strict)"("Val(Sgnl)"=w227) -> ()  [unwired: 2 in, 2 out]
      }
    }
    n781 = case shown="True" "Add Button" {
      tunnel: w180 -> [_ w226]
      frame False {
      }
      frame True {
        n782 = property on="X Step PV" class="DigNum (strict)"() -> ("Value"=w221:i32)  [unwired: 2 in, 2 out]
        n783 = property on="Y Step PV" class="DigNum (strict)"() -> ("Value"=w220:i32)  [unwired: 2 in, 2 out]
        n784 = property on="Z Step PV" class="DigNum (strict)"() -> ("Value"=w219:i32)  [unwired: 2 in, 2 out]
        n785 = property on="R Step PV" class="DigNum (strict)"() -> ("Value"=w218:i32)  [unwired: 2 in, 2 out]
        n786 = Build Array(w221, w220, w219, w218) -> (w224:i32[])
        n787 = Build Array (concatenate)(w226, "String") -> (w225:string[])
        n788 = property on="Preset positions" class="Ring (strict)"("Strings []"=w225) -> ()  [unwired: 2 in, 2 out]
        n789 = property on="Presets" class="Arr (strict)"() -> ("Value"=w223:i32[][])  [unwired: 2 in, 2 out]
        n790 = Build Array (concatenate)(w223, w224) -> (w217:i32[][])
        n791 = property on="Presets" class="Arr (strict)"("Val(Sgnl)"=w217) -> ()  [unwired: 2 in, 2 out]
      }
    }
    n792 = case shown="True" "Delete Button" {
      tunnel: w180 -> [_ w216]
      frame False {
      }
      frame True {
        n793 = property on="Preset positions" class="Ring (strict)"() -> ("Value"=w214:i32)  [unwired: 2 in, 2 out]
        n794 = property on="Presets" class="Arr (strict)"() -> ("Value"=w213:i32[][])  [unwired: 2 in, 2 out]
        n795 = Delete From Array(array=w216, index=w214) -> (array with subset deleted=w215:string[])  [unwired: 1 in, 1 out]
        n796 = property on="Preset positions" class="Ring (strict)"("Strings []"=w215) -> ()  [unwired: 2 in, 2 out]
        n797 = Delete From Array(array=w213, index (row)=w214) -> (array with subset deleted=w212:i32[][])  [unwired: 2 in, 1 out]
        n798 = property on="Presets" class="Arr (strict)"("Val(Sgnl)"=w212) -> ()  [unwired: 2 in, 2 out]
      }
    }
  }
  n799 = flat-sequence {
    tunnel: w23 -> [w1149]
    tunnel: w22 -> [w1147]
    tunnel: [w1144] -> w21
    frame #0 {
      n800 = call "mDrive Send Command.vi"("error in (no error)"=w1147, "Extra"="P", "Command"=T1."Print Parameter", "VISA resource name"=w1149) -> ("error out"=w1146:errorcluster, "read buffer"=w1153:string, "VISA resource name out"=w1148:refnum<visa-resource-name>)  [unwired: 3 in]
      n801 = call "mDrive Send Command.vi"("error in (no error)"=w1146, "Command"=T1."Stop", "VISA resource name"=w1148) -> ("error out"=w1155:errorcluster, "VISA resource name out"=w1156:refnum<visa-resource-name>)  [unwired: 4 in, 1 out]
      n802 = Decimal String To Number(string=w1153, offset=0) -> (number=w1145:i32)  [unwired: 1 in, 1 out]
      n803 = To Long Integer(number=w1145) -> (32bit integer=w1144:i32)
      n804 = VISA Close(VISA resource name=w1156, error in (no error)=w1155) -> ()  [unwired: 1 out]
    }
  }
  n805 = flat-sequence {
    tunnel: w21 -> [w1160]
    frame #0 {
      w1157 = 0
      n806 = Build Array(w1157, w1157, w1157, w1160) -> (w1158:i32[])
      n807 = call-poly <vilib>:"Write To Spreadsheet File.vi"("1D data"=w1158, "file path (dialog if empty)"=path "S:/SSE/IMS/POS.TXT") -> ()  [unwired: 6 in, 1 out]
    }
    frame #1 {
      n808 = property on="Presets" class="Arr (strict)"() -> ("Value"=w1167:i32[][])  [unwired: 2 in, 2 out]
      n809 = property on="Preset positions" class="Ring (strict)"() -> ("Strings []"=w1163:string[])  [unwired: 2 in, 2 out]
      n810 = Number To Decimal String(number=w1167) -> (decimal integer string=w1161:string[][])  [unwired: 1 in]
      n811 = Transpose 2D Array(2D array=w1161) -> (transposed array=w1162:string[][])
      n812 = Build Array (concatenate)(w1163, w1162) -> (w1164:string[][])
      n813 = Transpose 2D Array(2D array=w1164) -> (transposed array=w1165:string[][])
      n814 = call-poly <vilib>:"Write To Spreadsheet File.vi"("2D data"=w1165, "file path (dialog if empty)"=path "S:/SSE/IMS/PRESET.TXT") -> ()  [unwired: 6 in, 1 out]
    }
  }
